vi "HandleObservationAsync.vi"(8 "error in (no error)":errorcluster, 10 "Acquisition.lvclass In":refnum<class "Acquisition.lvclass">, 11 "S4ACS_GUI in":refnum<class "S4ACS_GUI.lvclass">) -> (0 "error out":errorcluster, 2 "Acquisition.lvclass Out":refnum<class "Acquisition.lvclass">, 3 "S4ACS_GUI out":refnum<class "S4ACS_GUI.lvclass">)   [LabVIEW 2018, in "S4ACS_GUI.lvclass"]
uses:
  S4ACS_GUI.lvclass
  Acquisition/Acquisition.lvclass
  S4ACS_GUI.lvclass/S4ACS_GUI.ctl
  Instrument/Instrument.lvclass/Instrument.ctl
  Device/Optics/Optics.lvclass/Optics.ctl
  Device/Optics/Opt_Selector/Opt_Selector.lvclass
  C:/Users/observer/Desktop/Sparc4GUI/SPARC4_GUI/Device/Optics/Optics.lvclass
  Instrument/Instrument.lvclass
  StateMachine/State Machine.lvclass
  SyncBox/Sync Box.lvclass
  Trigger/Trigger.lvclass
  Channel/Channel.lvclass
  Device/Optics/Optics.lvclass
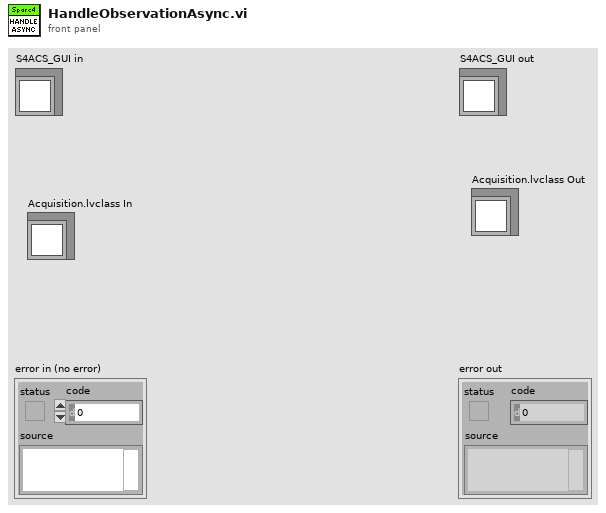
[diagram p1: front panel]
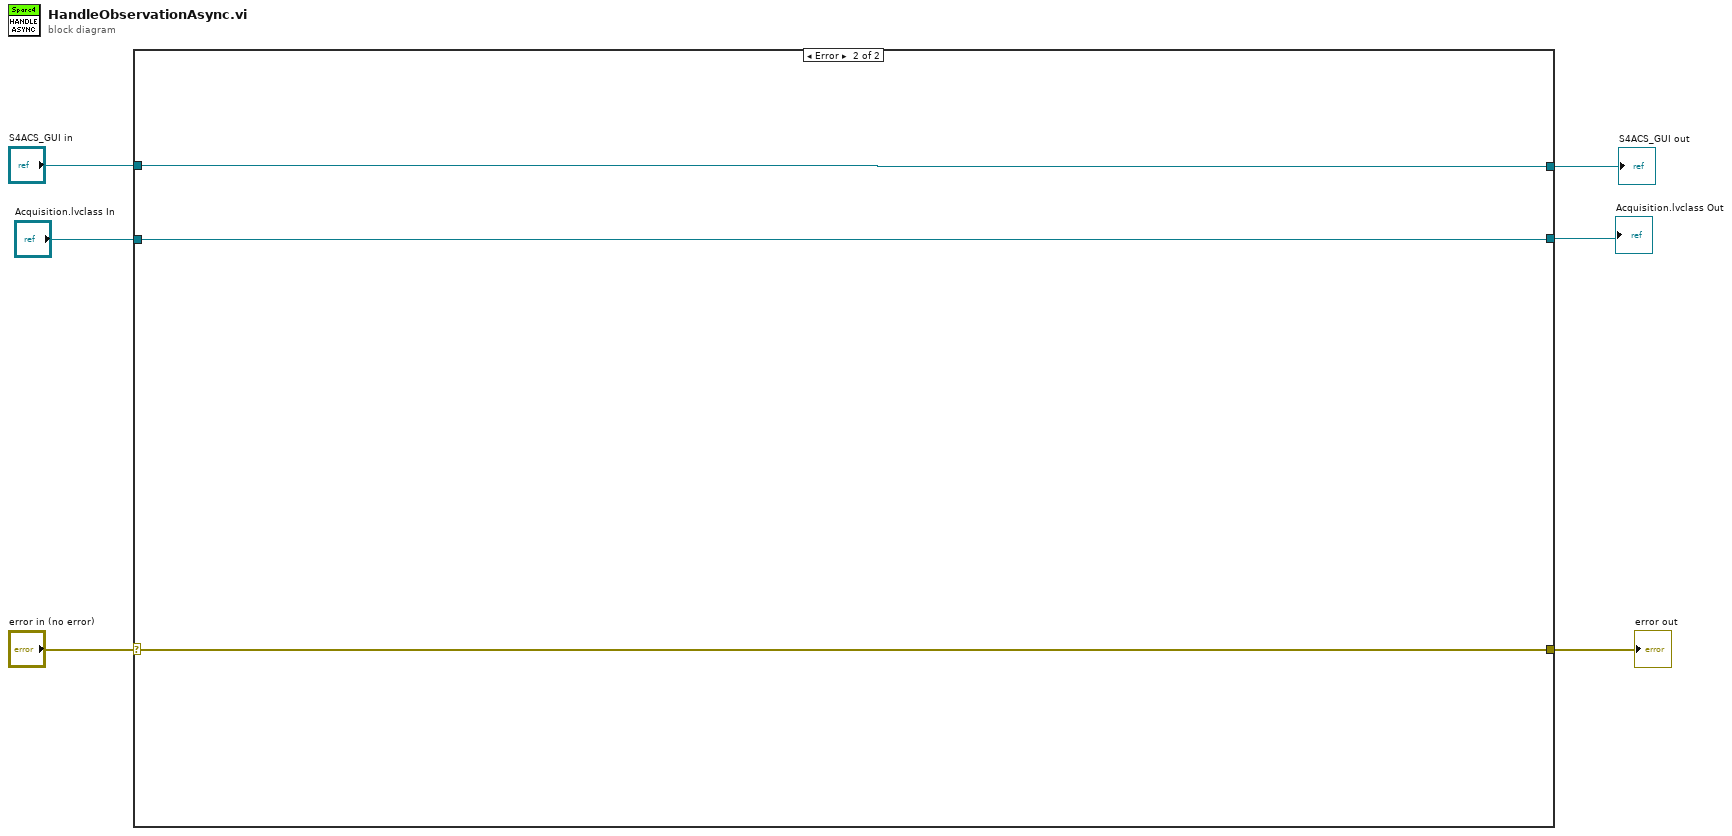
[diagram p0: block diagram]
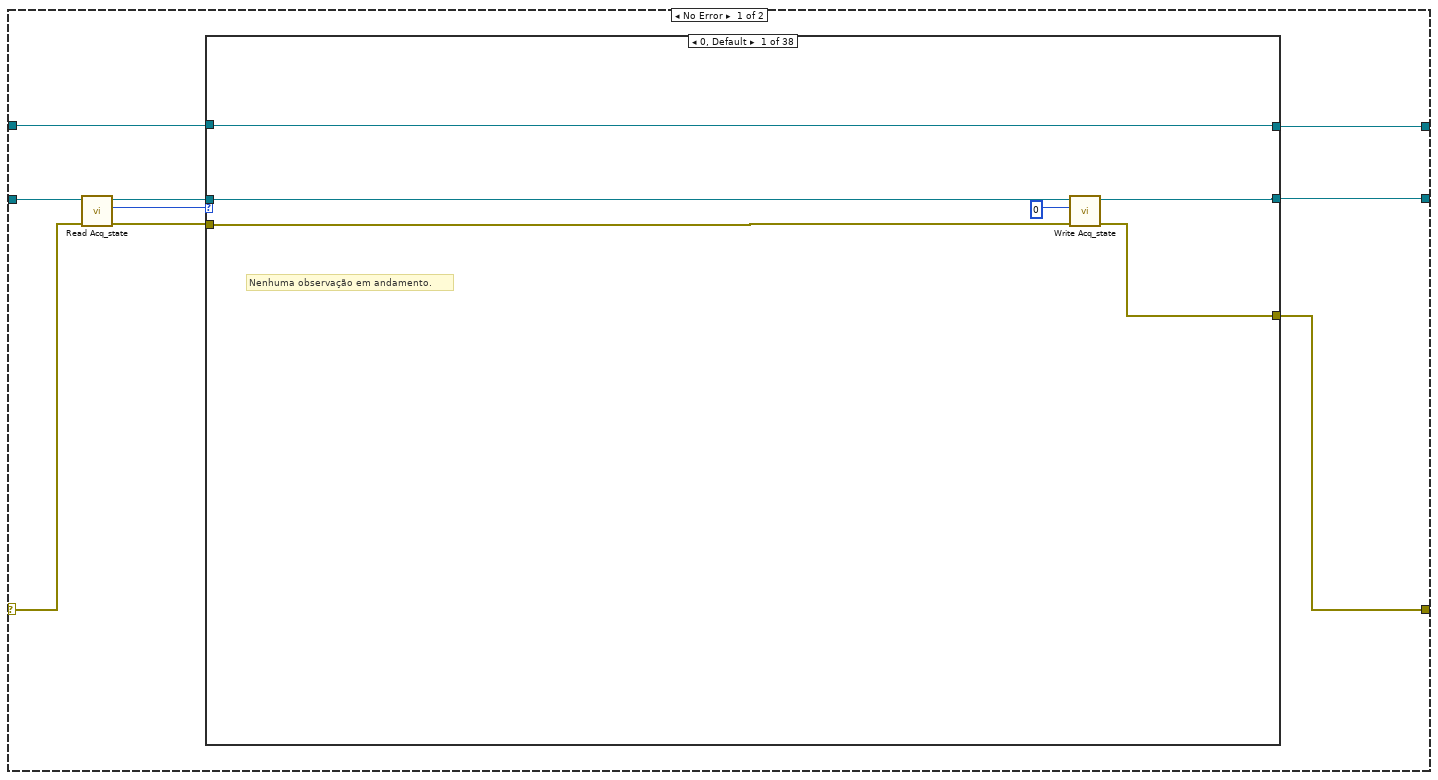
[diagram p2: hidden frame]
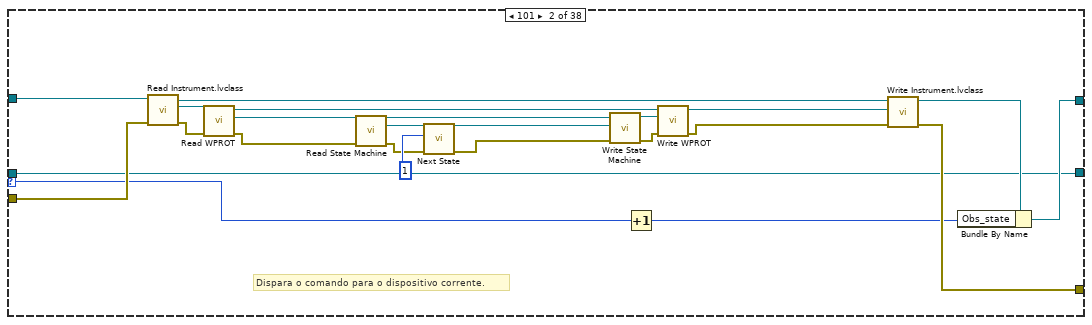
[diagram p3: hidden frame]
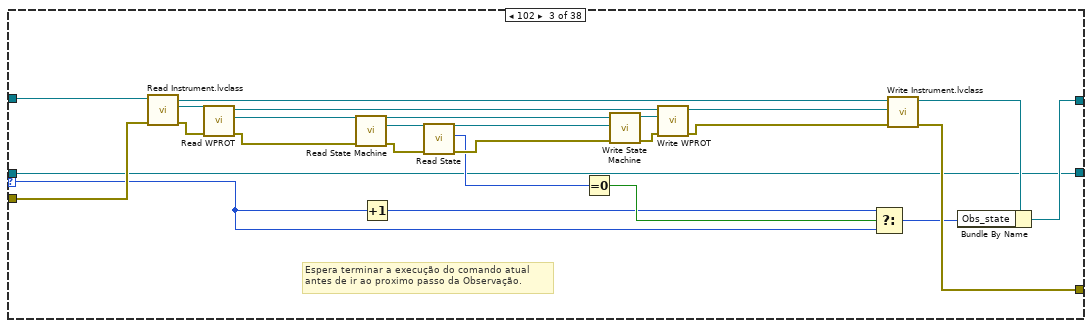
[diagram p4: hidden frame]
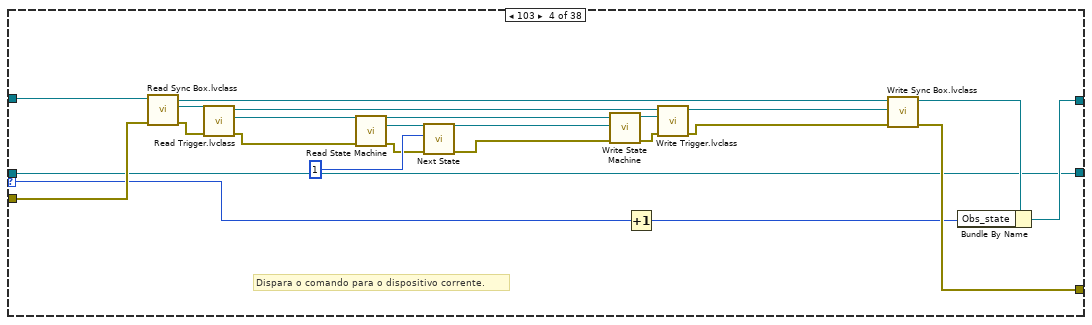
[diagram p5: hidden frame]
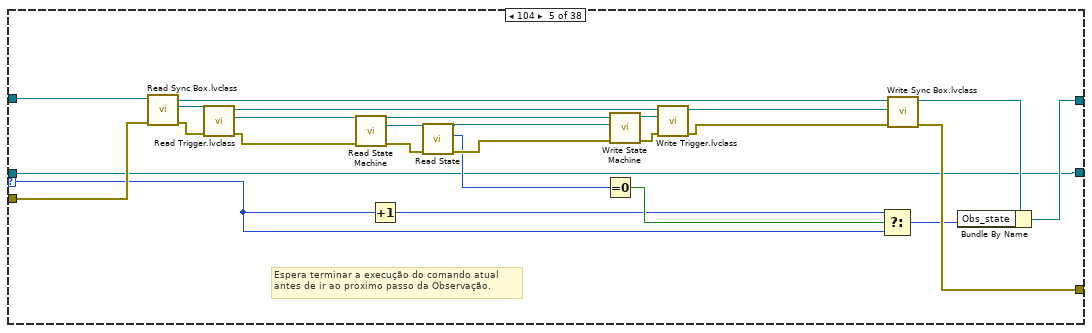
[diagram p6: hidden frame]
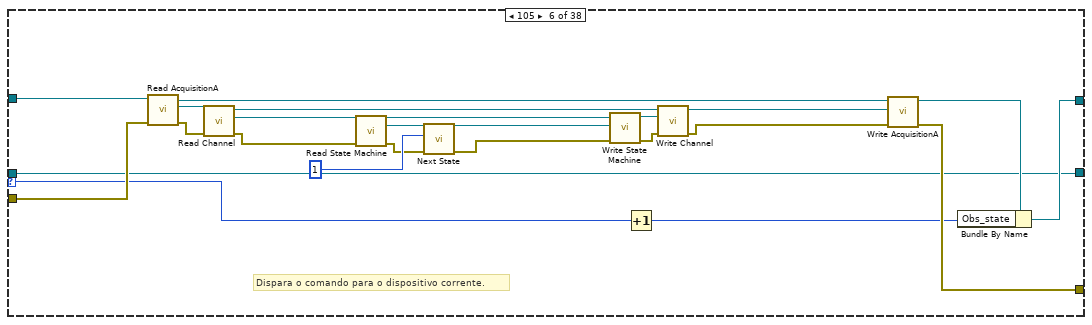
[diagram p7: hidden frame]
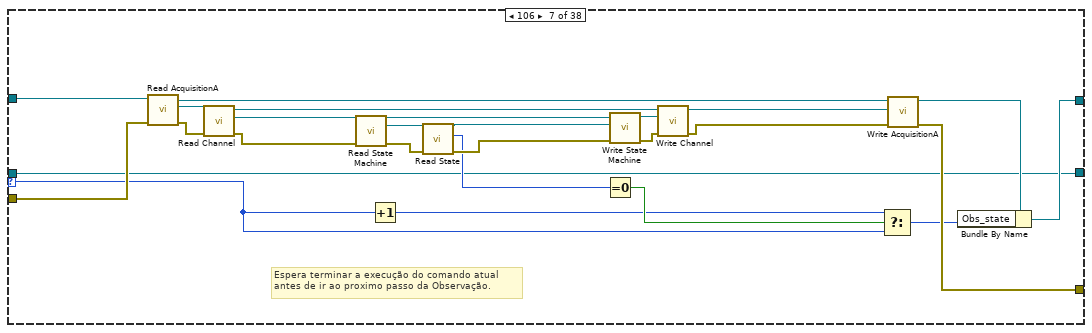
[diagram p8: hidden frame]
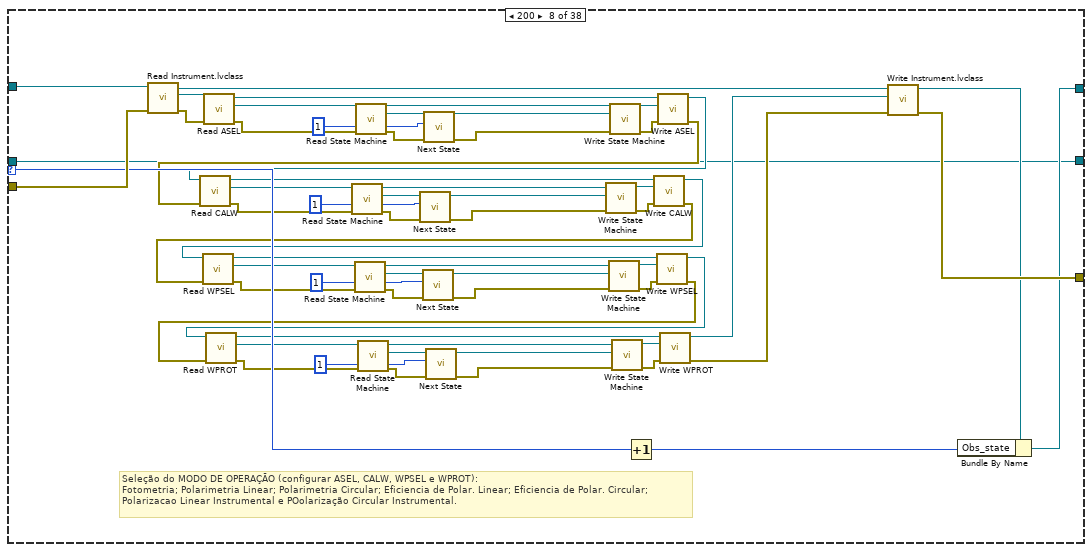
[diagram p9: hidden frame]
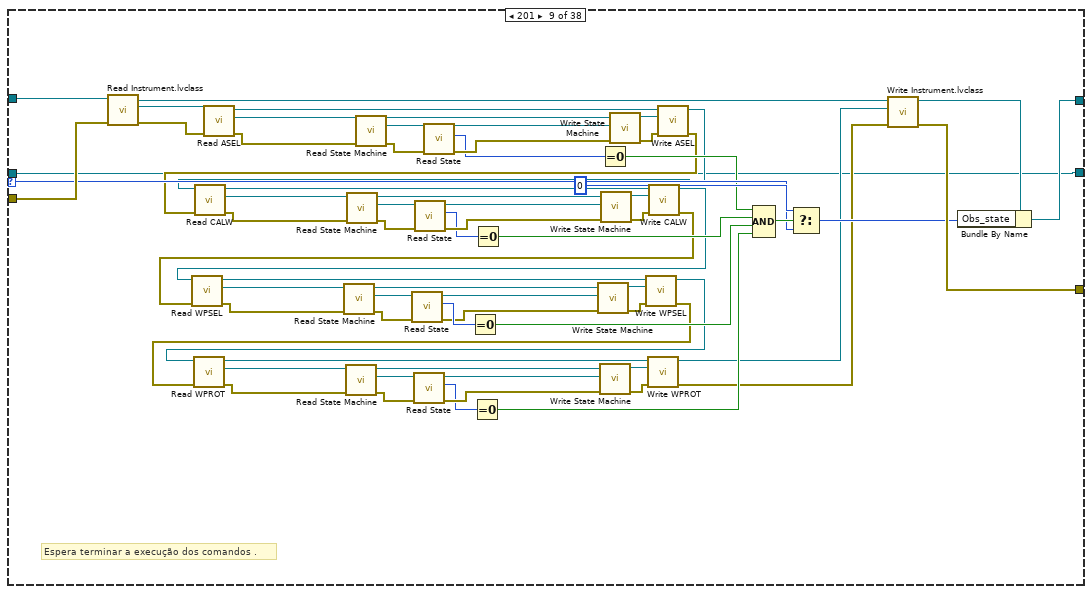
[diagram p10: hidden frame]
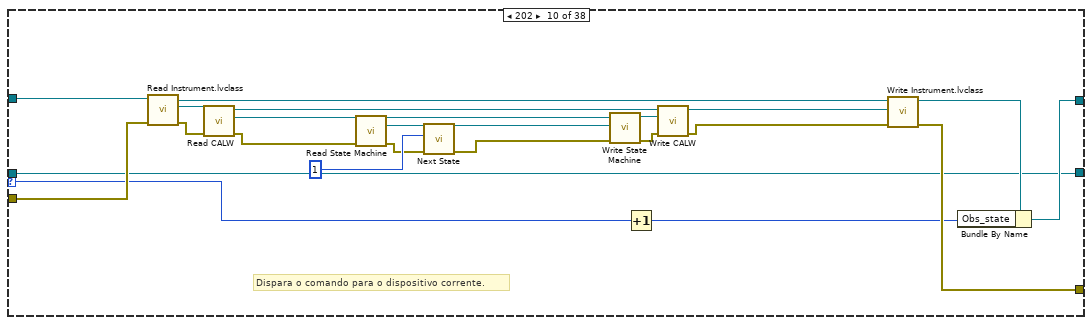
[diagram p11: hidden frame]
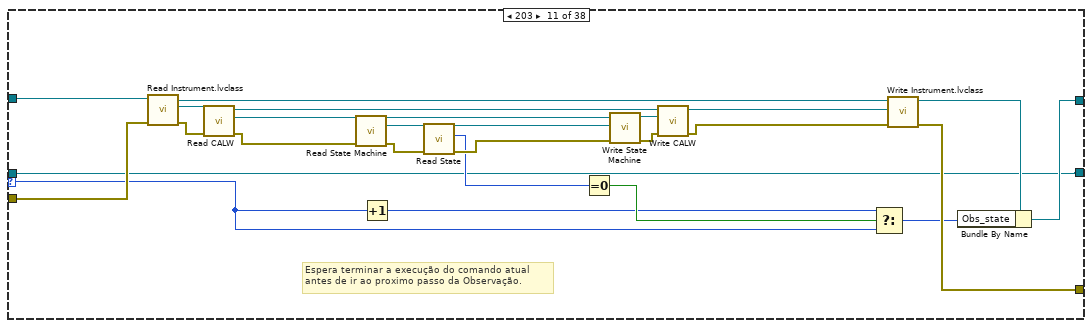
[diagram p12: hidden frame]
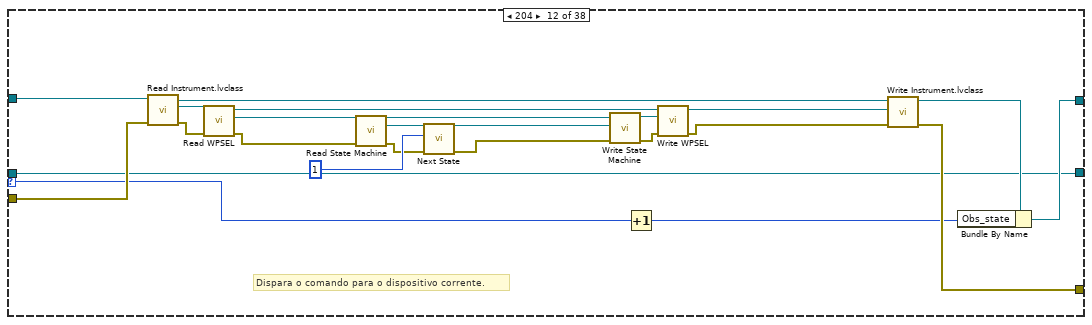
[diagram p13: hidden frame]
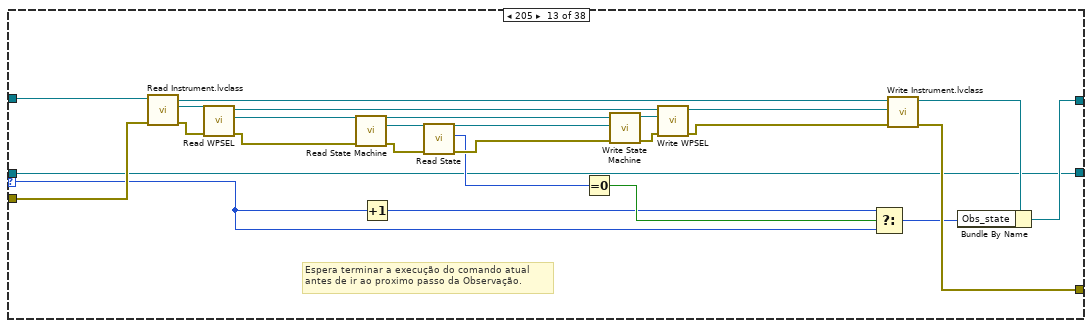
[diagram p14: hidden frame]
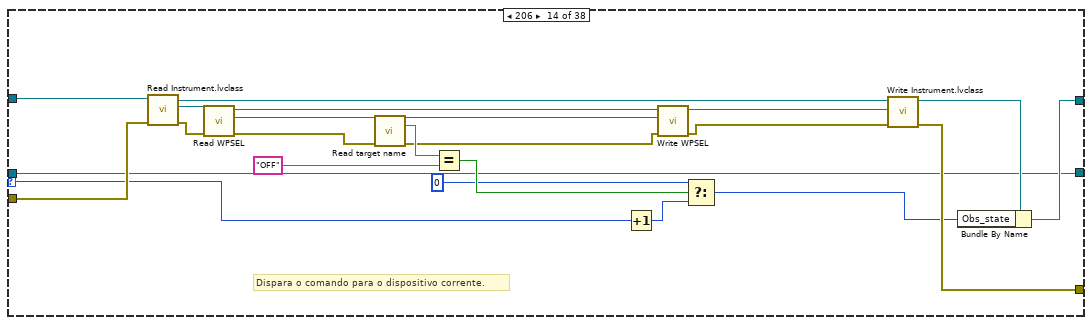
[diagram p15: hidden frame]
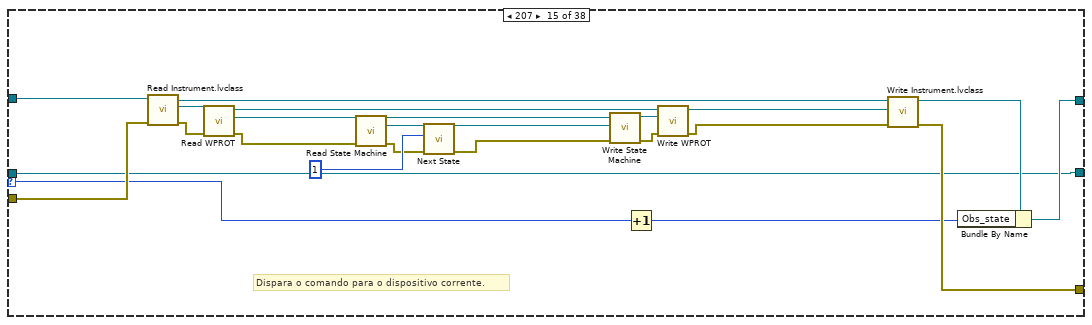
[diagram p16: hidden frame]
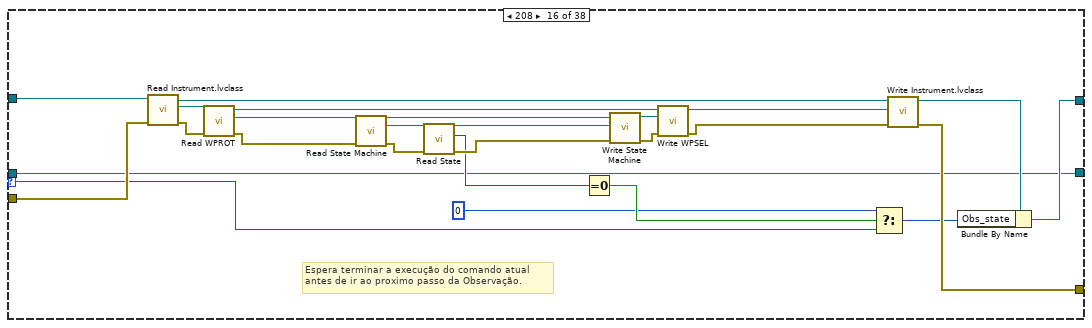
[diagram p17: hidden frame]
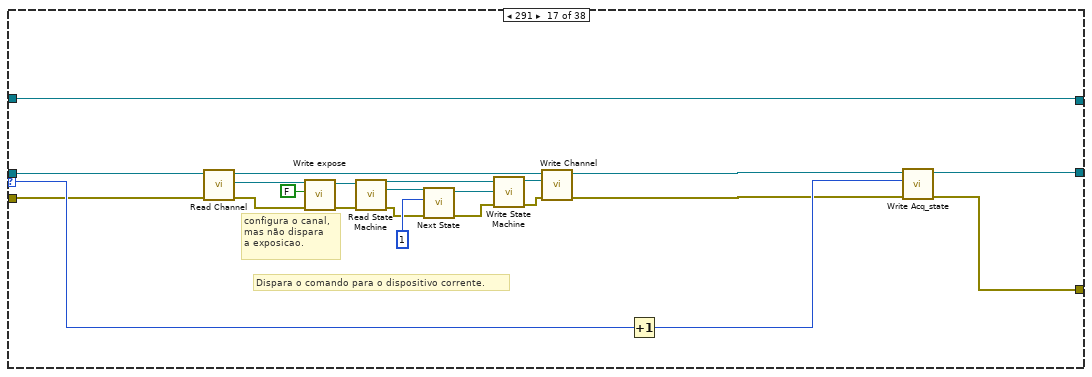
[diagram p18: hidden frame]
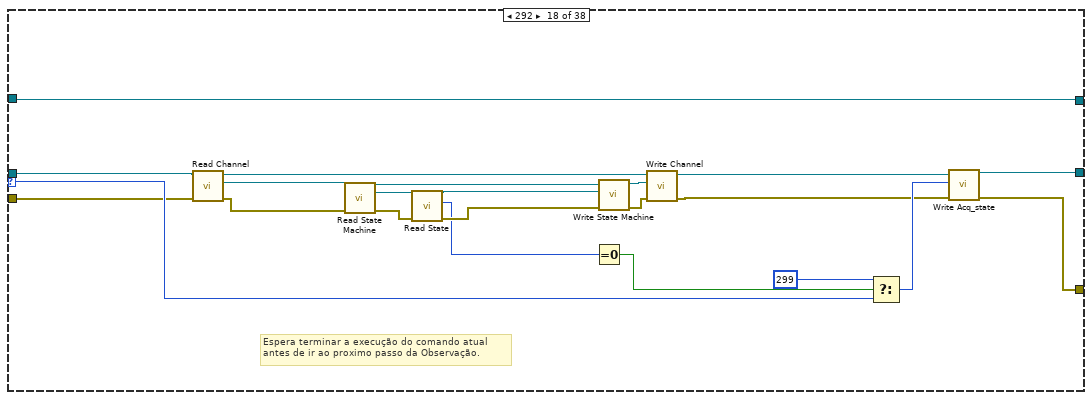
[diagram p19: hidden frame]
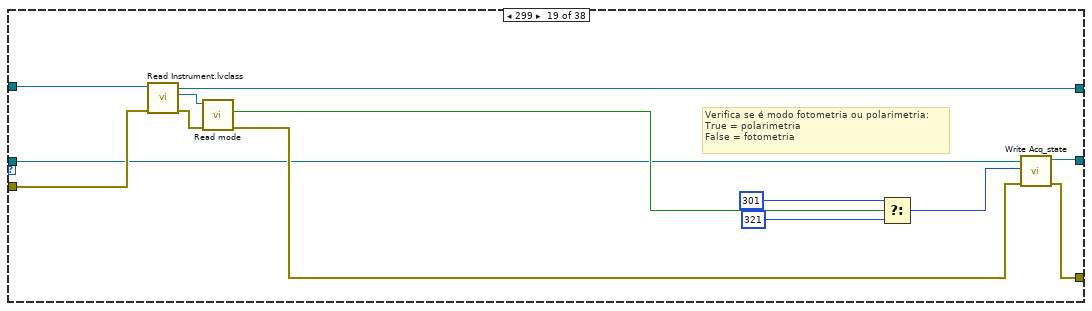
[diagram p20: hidden frame]
diagram:
  n1 = case shown="Error" "error in (no error)" {
    selector: "error in (no error)" -> [w9 w1155]
    tunnel: [w15 w1155] -> w5
    tunnel: [w14 w1154] -> w3
    tunnel: "S4ACS_GUI in" -> [w13 w1154]
    tunnel: "Acquisition.lvclass In" -> [w12 w1153]
    tunnel: [w7 w1153] -> w1
    frame No Error {
      n2 = call-dynamic "Read Acq_state.vi"("error in (no error)"=w9, "Acquisition in"=w12) -> ("error out"=w8:errorcluster, "Acq_state"=w10:u32, "Acquisition out"=w11:refnum<class "Acquisition.lvclass">)  [unwired: 7 in]
      n3 = case shown="0, Default" w10 {
        selector: w10 -> [_ w25 w48 w75 w98 w125 w148 w217 w281 w307 w330 w357 w380 w416 w430 w453 w492 w508 _ w570 w620 w644 w675 w718 w758 w774 w805 w845 w881 _ w931 w974 w1014 w1035 w1075 w1111 _ _]
        tunnel: w13 -> [w20 w39 w65 w89 w115 w139 w165 w231 w299 w321 w347 w371 w397 w420 w444 w470 w479 w506 w534 w572 w631 w657 w677 w730 w749 w787 w807 w857 w874 w903 w933 w986 w1002 w1037 w1087 w1104 w1135 w1152]
        tunnel: [w20 w23 w52 w73 w106 w123 w156 w215 w286 w305 w334 w355 w384 w415 w428 w457 w479 w506 w527 w537 w608 w643 w674 w712 w749 w773 w804 w844 w874 w903 w930 w973 w1002 w1029 w1074 w1104 w1135 w1152] -> w14
        tunnel: w8 -> [w19 w38 w64 w88 w114 w138 w164 w230 w298 w320 w346 w370 w396 w419 w443 w469 w483 w500 w533 w571 w630 w656 w676 w729 w751 w786 w806 w856 w878 w910 w932 w985 w1007 w1036 w1086 w1103 w1139 w1151]
        tunnel: [w16 w37 w63 w87 w113 w137 w163 w229 w297 w319 w345 w369 w395 w418 w442 w468 w477 w501 w523 w536 w610 w639 w670 w707 w745 w769 w799 w841 w872 w896 w925 w970 w1001 w1026 w1071 w1107 w1125 w1151] -> w15
        tunnel: w11 -> [w18 w22 w46 w72 w96 w122 w146 w172 w235 w304 w328 w354 w378 w404 w427 w451 w484 w507 w524 w539 w612 w638 w669 w709 w752 w768 w800 w834 w879 w909 w926 w969 w1008 w1024 w1064 w1102 w1140 w1150]
        tunnel: [w17 w22 w46 w72 w96 w122 w146 w172 w235 w304 w328 w354 w378 w404 w427 w451 w480 w502 w522 w535 w609 w640 w671 w708 w746 w772 w803 w842 w873 w897 w929 w972 w1006 w1025 w1072 w1109 w1131 w1150] -> w7
        frame 0, Default {
          # "Nenhuma observação em andamento."
          n4 = call-dynamic "Write Acq_state.vi"("error in (no error)"=w19, "Acq_state"=u32 0 ("Obs_state"), "Acquisition in"=w18) -> ("error out"=w16:errorcluster, "Acquisition out"=w17:refnum<class "Acquisition.lvclass">)  [unwired: 7 in]
        }
        frame 101 {
          # "Dispara o comando para o dispositivo corrente."
          n5 = call "Read Instrument.lvclass.vi"("error in (no error)"=w38, "S4ACS_GUI in"=w39) -> ("error out"=w44:errorcluster, "Instrument.lvclass"=w45:refnum<class "Instrument.lvclass">, "S4ACS_GUI out"=w41:refnum<class "S4ACS_GUI.lvclass">)  [unwired: 7 in]
          n6 = call "Read WPROT.vi"("error in (no error)"=w44, "Instrument in"=w45) -> ("error out"=w31:errorcluster, "Opt_Selector.lvclass"=w30:refnum<class "Opt_Selector.lvclass">, "Instrument out"=w43:refnum<class "Instrument.lvclass">)  [unwired: 7 in]
          n7 = call-dynamic "Read State Machine.vi"("error in (no error)"=w31, "Device in"=w30) -> ("error out"=w34:errorcluster, "State Machine.lvclass"=w36:refnum<class "State Machine.lvclass">, "Device out"=w28:refnum<class "Opt_Selector.lvclass">)  [unwired: 7 in]
          n8 = call "Next State.vi"("error in (no error)"=w34, "New_State"=1, "State Machine in"=w36) -> ("error out"=w33:errorcluster, "State Machine out"=w32:refnum<class "State Machine.lvclass">)  [unwired: 7 in]
          n9 = call-dynamic "Write State Machine.vi"("error in (no error)"=w33, "State Machine.lvclass"=w32, "Device in"=w28) -> ("error out"=w27:errorcluster, "Device out"=w29:refnum<class "Opt_Selector.lvclass">)  [unwired: 7 in]
          n10 = Increment(x=w25) -> (x+1=w24:u32)
          n11 = call "Write WPROT.vi"("error in (no error)"=w27, "Opt_Selector.lvclass"=w29, "Instrument in"=w43) -> ("error out"=w40:errorcluster, "Instrument out"=w42:refnum<class "Instrument.lvclass">)  [unwired: 7 in]
          n12 = call "Write Instrument.lvclass.vi"("error in (no error)"=w40, "Instrument.lvclass"=w42, "S4ACS_GUI in"=w41) -> ("error out"=w37:errorcluster, "S4ACS_GUI out"=w26:refnum<class "S4ACS_GUI.lvclass">)  [unwired: 7 in]
          n13 = Bundle By Name(cluster=w26, "Obs_state"=w24) -> (w23:refnum<class "S4ACS_GUI.lvclass">)
        }
        frame 102 {
          # "Espera terminar a execução do comando atual \nantes de ir ao proximo passo da Observação."
          n14 = call "Read Instrument.lvclass.vi"("error in (no error)"=w64, "S4ACS_GUI in"=w65) -> ("error out"=w70:errorcluster, "Instrument.lvclass"=w71:refnum<class "Instrument.lvclass">, "S4ACS_GUI out"=w67:refnum<class "S4ACS_GUI.lvclass">)  [unwired: 7 in]
          n15 = call "Read WPROT.vi"("error in (no error)"=w70, "Instrument in"=w71) -> ("error out"=w58:errorcluster, "Opt_Selector.lvclass"=w57:refnum<class "Opt_Selector.lvclass">, "Instrument out"=w69:refnum<class "Instrument.lvclass">)  [unwired: 7 in]
          n16 = call-dynamic "Read State Machine.vi"("error in (no error)"=w58, "Device in"=w57) -> ("error out"=w61:errorcluster, "State Machine.lvclass"=w62:refnum<class "State Machine.lvclass">, "Device out"=w55:refnum<class "Opt_Selector.lvclass">)  [unwired: 7 in]
          n17 = Increment(x=w48) -> (x+1=w47:u32)
          n18 = call-dynamic "Read State.vi"("error in (no error)"=w61, "State Machine in"=w62) -> ("error out"=w60:errorcluster, "State"=w50:i32, "State Machine out"=w59:refnum<class "State Machine.lvclass">)  [unwired: 7 in]
          n19 = Equal To 0?(x=w50) -> (x = 0?=w51:bool)
          n20 = call-dynamic "Write State Machine.vi"("error in (no error)"=w60, "State Machine.lvclass"=w59, "Device in"=w55) -> ("error out"=w54:errorcluster, "Device out"=w56:refnum<class "Opt_Selector.lvclass">)  [unwired: 7 in]
          n21 = call "Write WPROT.vi"("error in (no error)"=w54, "Opt_Selector.lvclass"=w56, "Instrument in"=w69) -> ("error out"=w66:errorcluster, "Instrument out"=w68:refnum<class "Instrument.lvclass">)  [unwired: 7 in]
          n22 = Select(t=w47, s=w51, f=w48) -> (s? t:f=w49:u32)
          n23 = call "Write Instrument.lvclass.vi"("error in (no error)"=w66, "Instrument.lvclass"=w68, "S4ACS_GUI in"=w67) -> ("error out"=w63:errorcluster, "S4ACS_GUI out"=w53:refnum<class "S4ACS_GUI.lvclass">)  [unwired: 7 in]
          n24 = Bundle By Name(cluster=w53, "Obs_state"=w49) -> (w52:refnum<class "S4ACS_GUI.lvclass">)
        }
        frame 103 {
          # "Dispara o comando para o dispositivo corrente."
          n25 = call-dynamic "Read Sync Box.lvclass.vi"("error in (no error)"=w88, "SPARC4_AC in"=w89) -> ("error out"=w94:errorcluster, "Sync Box.lvclass"=w95:refnum<class "Sync Box.lvclass">, "SPARC4_AC out"=w91:refnum<class "S4ACS_GUI.lvclass">)  [unwired: 7 in]
          n26 = call-dynamic "Read Trigger.lvclass.vi"("error in (no error)"=w94, "Sync Box in"=w95) -> ("error out"=w81:errorcluster, "Trigger.lvclass"=w80:refnum<class "Trigger.lvclass">, "Sync Box out"=w93:refnum<class "Sync Box.lvclass">)  [unwired: 7 in]
          n27 = call-dynamic "Read State Machine.vi"("error in (no error)"=w81, "Device in"=w80) -> ("error out"=w84:errorcluster, "State Machine.lvclass"=w86:refnum<class "State Machine.lvclass">, "Device out"=w78:refnum<class "Trigger.lvclass">)  [unwired: 7 in]
          n28 = call "Next State.vi"("error in (no error)"=w84, "New_State"=1, "State Machine in"=w86) -> ("error out"=w83:errorcluster, "State Machine out"=w82:refnum<class "State Machine.lvclass">)  [unwired: 7 in]
          n29 = call-dynamic "Write State Machine.vi"("error in (no error)"=w83, "State Machine.lvclass"=w82, "Device in"=w78) -> ("error out"=w77:errorcluster, "Device out"=w79:refnum<class "Trigger.lvclass">)  [unwired: 7 in]
          n30 = Increment(x=w75) -> (x+1=w74:u32)
          n31 = call-dynamic "Write Trigger.lvclass.vi"("error in (no error)"=w77, "Trigger.lvclass"=w79, "Sync Box in"=w93) -> ("error out"=w90:errorcluster, "Sync Box out"=w92:refnum<class "Sync Box.lvclass">)  [unwired: 7 in]
          n32 = call-dynamic "Write Sync Box.lvclass.vi"("error in (no error)"=w90, "Sync Box.lvclass"=w92, "SPARC4_AC in"=w91) -> ("error out"=w87:errorcluster, "SPARC4_AC out"=w76:refnum<class "S4ACS_GUI.lvclass">)  [unwired: 7 in]
          n33 = Bundle By Name(cluster=w76, "Obs_state"=w74) -> (w73:refnum<class "S4ACS_GUI.lvclass">)
        }
        frame 104 {
          # "Espera terminar a execução do comando atual \nantes de ir ao proximo passo da Observação."
          n34 = call-dynamic "Read Sync Box.lvclass.vi"("error in (no error)"=w114, "SPARC4_AC in"=w115) -> ("error out"=w120:errorcluster, "Sync Box.lvclass"=w121:refnum<class "Sync Box.lvclass">, "SPARC4_AC out"=w117:refnum<class "S4ACS_GUI.lvclass">)  [unwired: 7 in]
          n35 = call-dynamic "Read Trigger.lvclass.vi"("error in (no error)"=w120, "Sync Box in"=w121) -> ("error out"=w112:errorcluster, "Trigger.lvclass"=w111:refnum<class "Trigger.lvclass">, "Sync Box out"=w119:refnum<class "Sync Box.lvclass">)  [unwired: 7 in]
          n36 = call-dynamic "Read State Machine.vi"("error in (no error)"=w112, "Device in"=w111) -> ("error out"=w103:errorcluster, "State Machine.lvclass"=w105:refnum<class "State Machine.lvclass">, "Device out"=w109:refnum<class "Trigger.lvclass">)  [unwired: 7 in]
          n37 = Increment(x=w98) -> (x+1=w100:u32)
          n38 = call-dynamic "Read State.vi"("error in (no error)"=w103, "State Machine in"=w105) -> ("error out"=w102:errorcluster, "State"=w97:i32, "State Machine out"=w104:refnum<class "State Machine.lvclass">)  [unwired: 7 in]
          n39 = Equal To 0?(x=w97) -> (x = 0?=w101:bool)
          n40 = call-dynamic "Write State Machine.vi"("error in (no error)"=w102, "State Machine.lvclass"=w104, "Device in"=w109) -> ("error out"=w108:errorcluster, "Device out"=w110:refnum<class "Trigger.lvclass">)  [unwired: 7 in]
          n41 = call-dynamic "Write Trigger.lvclass.vi"("error in (no error)"=w108, "Trigger.lvclass"=w110, "Sync Box in"=w119) -> ("error out"=w116:errorcluster, "Sync Box out"=w118:refnum<class "Sync Box.lvclass">)  [unwired: 7 in]
          n42 = Select(t=w100, s=w101, f=w98) -> (s? t:f=w99:u32)
          n43 = call-dynamic "Write Sync Box.lvclass.vi"("error in (no error)"=w116, "Sync Box.lvclass"=w118, "SPARC4_AC in"=w117) -> ("error out"=w113:errorcluster, "SPARC4_AC out"=w107:refnum<class "S4ACS_GUI.lvclass">)  [unwired: 7 in]
          n44 = Bundle By Name(cluster=w107, "Obs_state"=w99) -> (w106:refnum<class "S4ACS_GUI.lvclass">)
        }
        frame 105 {
          # "Dispara o comando para o dispositivo corrente."
          n45 = call-dynamic "Read AcquisitionA.vi"("error in (no error)"=w138, "S4ACS_GUI in"=w139) -> ("error out"=w144:errorcluster, "Acquisition.lvclass"=w145:refnum<class "Acquisition.lvclass">, "S4ACS_GUI out"=w141:refnum<class "S4ACS_GUI.lvclass">)  [unwired: 7 in]
          n46 = call-dynamic "Read Channel.vi"("error in (no error)"=w144, "Acquisition in"=w145) -> ("error out"=w131:errorcluster, "Channel.lvclass"=w130:refnum<class "Channel.lvclass">, "Acquisition out"=w143:refnum<class "Acquisition.lvclass">)  [unwired: 7 in]
          n47 = call-dynamic "Read State Machine.vi"("error in (no error)"=w131, "Device in"=w130) -> ("error out"=w134:errorcluster, "State Machine.lvclass"=w136:refnum<class "State Machine.lvclass">, "Device out"=w128:refnum<class "Channel.lvclass">)  [unwired: 7 in]
          n48 = call "Next State.vi"("error in (no error)"=w134, "New_State"=1, "State Machine in"=w136) -> ("error out"=w133:errorcluster, "State Machine out"=w132:refnum<class "State Machine.lvclass">)  [unwired: 7 in]
          n49 = call-dynamic "Write State Machine.vi"("error in (no error)"=w133, "State Machine.lvclass"=w132, "Device in"=w128) -> ("error out"=w127:errorcluster, "Device out"=w129:refnum<class "Channel.lvclass">)  [unwired: 7 in]
          n50 = Increment(x=w125) -> (x+1=w124:u32)
          n51 = call-dynamic "Write Channel.vi"("error in (no error)"=w127, "Channel.lvclass"=w129, "Acquisition in"=w143) -> ("error out"=w140:errorcluster, "Acquisition out"=w142:refnum<class "Acquisition.lvclass">)  [unwired: 7 in]
          n52 = call-dynamic "Write AcquisitionA.vi"("error in (no error)"=w140, "Acquisition.lvclass"=w142, "S4ACS_GUI in"=w141) -> ("error out"=w137:errorcluster, "S4ACS_GUI out"=w126:refnum<class "S4ACS_GUI.lvclass">)  [unwired: 7 in]
          n53 = Bundle By Name(cluster=w126, "Obs_state"=w124) -> (w123:refnum<class "S4ACS_GUI.lvclass">)
        }
        frame 106 {
          # "Espera terminar a execução do comando atual \nantes de ir ao proximo passo da Observação."
          n54 = call-dynamic "Read AcquisitionA.vi"("error in (no error)"=w164, "S4ACS_GUI in"=w165) -> ("error out"=w170:errorcluster, "Acquisition.lvclass"=w171:refnum<class "Acquisition.lvclass">, "S4ACS_GUI out"=w167:refnum<class "S4ACS_GUI.lvclass">)  [unwired: 7 in]
          n55 = call-dynamic "Read Channel.vi"("error in (no error)"=w170, "Acquisition in"=w171) -> ("error out"=w162:errorcluster, "Channel.lvclass"=w161:refnum<class "Channel.lvclass">, "Acquisition out"=w169:refnum<class "Acquisition.lvclass">)  [unwired: 7 in]
          n56 = call-dynamic "Read State Machine.vi"("error in (no error)"=w162, "Device in"=w161) -> ("error out"=w153:errorcluster, "State Machine.lvclass"=w155:refnum<class "State Machine.lvclass">, "Device out"=w159:refnum<class "Channel.lvclass">)  [unwired: 7 in]
          n57 = Increment(x=w148) -> (x+1=w150:u32)
          n58 = call-dynamic "Read State.vi"("error in (no error)"=w153, "State Machine in"=w155) -> ("error out"=w152:errorcluster, "State"=w147:i32, "State Machine out"=w154:refnum<class "State Machine.lvclass">)  [unwired: 7 in]
          n59 = Equal To 0?(x=w147) -> (x = 0?=w151:bool)
          n60 = call-dynamic "Write State Machine.vi"("error in (no error)"=w152, "State Machine.lvclass"=w154, "Device in"=w159) -> ("error out"=w158:errorcluster, "Device out"=w160:refnum<class "Channel.lvclass">)  [unwired: 7 in]
          n61 = call-dynamic "Write Channel.vi"("error in (no error)"=w158, "Channel.lvclass"=w160, "Acquisition in"=w169) -> ("error out"=w166:errorcluster, "Acquisition out"=w168:refnum<class "Acquisition.lvclass">)  [unwired: 7 in]
          n62 = Select(t=w150, s=w151, f=w148) -> (s? t:f=w149:u32)
          n63 = call-dynamic "Write AcquisitionA.vi"("error in (no error)"=w166, "Acquisition.lvclass"=w168, "S4ACS_GUI in"=w167) -> ("error out"=w163:errorcluster, "S4ACS_GUI out"=w157:refnum<class "S4ACS_GUI.lvclass">)  [unwired: 7 in]
          n64 = Bundle By Name(cluster=w157, "Obs_state"=w149) -> (w156:refnum<class "S4ACS_GUI.lvclass">)
        }
        frame 200 {
          # "Seleção do MODO DE OPERAÇÃO (configurar ASEL, CALW, WPSEL e WPROT): \nFotometria; Polarimetria Linear; Polarimetria Circular; Eficiencia de Polar. Linear; Eficiencia de Polar. Circular;\nPolarizacao Linear Instrumental e POolarização Circular Instrumental."
          n65 = call "Read Instrument.lvclass.vi"("error in (no error)"=w230, "S4ACS_GUI in"=w231) -> ("error out"=w234:errorcluster, "Instrument.lvclass"=w194:refnum<class "Instrument.lvclass">, "S4ACS_GUI out"=w232:refnum<class "S4ACS_GUI.lvclass">)  [unwired: 7 in]
          n66 = call "Read ASEL.vi"("error in (no error)"=w234, "Instrument in"=w194) -> ("error out"=w223:errorcluster, "Opt_Selector.lvclass"=w222:refnum<class "Opt_Selector.lvclass">, "Instrument out"=w233:refnum<class "Instrument.lvclass">)  [unwired: 7 in]
          n67 = call-dynamic "Read State Machine.vi"("error in (no error)"=w223, "Device in"=w222) -> ("error out"=w226:errorcluster, "State Machine.lvclass"=w228:refnum<class "State Machine.lvclass">, "Device out"=w220:refnum<class "Opt_Selector.lvclass">)  [unwired: 7 in]
          n68 = call "Next State.vi"("error in (no error)"=w226, "New_State"=1, "State Machine in"=w228) -> ("error out"=w225:errorcluster, "State Machine out"=w224:refnum<class "State Machine.lvclass">)  [unwired: 7 in]
          n69 = call-dynamic "Write State Machine.vi"("error in (no error)"=w225, "State Machine.lvclass"=w224, "Device in"=w220) -> ("error out"=w219:errorcluster, "Device out"=w221:refnum<class "Opt_Selector.lvclass">)  [unwired: 7 in]
          n70 = Increment(x=w217) -> (x+1=w216:u32)
          n71 = call "Write ASEL.vi"("error in (no error)"=w219, "Opt_Selector.lvclass"=w221, "Instrument in"=w233) -> ("error out"=w175:errorcluster, "Instrument out"=w193:refnum<class "Instrument.lvclass">)  [unwired: 7 in]
          n72 = call "Read CALW.vi"("error in (no error)"=w175, "Instrument in"=w193) -> ("error out"=w210:errorcluster, "Opt_Selector.lvclass"=w211:refnum<class "Opt_Selector.lvclass">, "Instrument out"=w192:refnum<class "Instrument.lvclass">)  [unwired: 7 in]
          n73 = call-dynamic "Read State Machine.vi"("error in (no error)"=w210, "Device in"=w211) -> ("error out"=w207:errorcluster, "State Machine.lvclass"=w205:refnum<class "State Machine.lvclass">, "Device out"=w213:refnum<class "Opt_Selector.lvclass">)  [unwired: 7 in]
          n74 = call "Next State.vi"("error in (no error)"=w207, "New_State"=1, "State Machine in"=w205) -> ("error out"=w208:errorcluster, "State Machine out"=w209:refnum<class "State Machine.lvclass">)  [unwired: 7 in]
          n75 = call-dynamic "Write State Machine.vi"("error in (no error)"=w208, "State Machine.lvclass"=w209, "Device in"=w213) -> ("error out"=w214:errorcluster, "Device out"=w212:refnum<class "Opt_Selector.lvclass">)  [unwired: 7 in]
          n76 = call "Write CALW.vi"("error in (no error)"=w214, "Opt_Selector.lvclass"=w212, "Instrument in"=w192) -> ("error out"=w174:errorcluster, "Instrument out"=w191:refnum<class "Instrument.lvclass">)  [unwired: 7 in]
          n77 = call "Read WPSEL.vi"("error in (no error)"=w174, "Instrument in"=w191) -> ("error out"=w199:errorcluster, "Opt_Selector.lvclass"=w198:refnum<class "Opt_Selector.lvclass">, "Instrument out"=w190:refnum<class "Instrument.lvclass">)  [unwired: 7 in]
          n78 = call-dynamic "Read State Machine.vi"("error in (no error)"=w199, "Device in"=w198) -> ("error out"=w202:errorcluster, "State Machine.lvclass"=w204:refnum<class "State Machine.lvclass">, "Device out"=w196:refnum<class "Opt_Selector.lvclass">)  [unwired: 7 in]
          n79 = call "Next State.vi"("error in (no error)"=w202, "New_State"=1, "State Machine in"=w204) -> ("error out"=w201:errorcluster, "State Machine out"=w200:refnum<class "State Machine.lvclass">)  [unwired: 7 in]
          n80 = call-dynamic "Write State Machine.vi"("error in (no error)"=w201, "State Machine.lvclass"=w200, "Device in"=w196) -> ("error out"=w195:errorcluster, "Device out"=w197:refnum<class "Opt_Selector.lvclass">)  [unwired: 7 in]
          n81 = call "Write WPSEL.vi"("error in (no error)"=w195, "Opt_Selector.lvclass"=w197, "Instrument in"=w190) -> ("error out"=w173:errorcluster, "Instrument out"=w179:refnum<class "Instrument.lvclass">)  [unwired: 7 in]
          n82 = call "Read WPROT.vi"("error in (no error)"=w173, "Instrument in"=w179) -> ("error out"=w185:errorcluster, "Opt_Selector.lvclass"=w186:refnum<class "Opt_Selector.lvclass">, "Instrument out"=w178:refnum<class "Instrument.lvclass">)  [unwired: 7 in]
          n83 = call-dynamic "Read State Machine.vi"("error in (no error)"=w185, "Device in"=w186) -> ("error out"=w182:errorcluster, "State Machine.lvclass"=w180:refnum<class "State Machine.lvclass">, "Device out"=w188:refnum<class "Opt_Selector.lvclass">)  [unwired: 7 in]
          n84 = call "Next State.vi"("error in (no error)"=w182, "New_State"=1, "State Machine in"=w180) -> ("error out"=w183:errorcluster, "State Machine out"=w184:refnum<class "State Machine.lvclass">)  [unwired: 7 in]
          n85 = call-dynamic "Write State Machine.vi"("error in (no error)"=w183, "State Machine.lvclass"=w184, "Device in"=w188) -> ("error out"=w189:errorcluster, "Device out"=w187:refnum<class "Opt_Selector.lvclass">)  [unwired: 7 in]
          n86 = call "Write WPROT.vi"("error in (no error)"=w189, "Opt_Selector.lvclass"=w187, "Instrument in"=w178) -> ("error out"=w176:errorcluster, "Instrument out"=w177:refnum<class "Instrument.lvclass">)  [unwired: 7 in]
          n87 = call "Write Instrument.lvclass.vi"("error in (no error)"=w176, "Instrument.lvclass"=w177, "S4ACS_GUI in"=w232) -> ("error out"=w229:errorcluster, "S4ACS_GUI out"=w218:refnum<class "S4ACS_GUI.lvclass">)  [unwired: 7 in]
          n88 = Bundle By Name(cluster=w218, "Obs_state"=w216) -> (w215:refnum<class "S4ACS_GUI.lvclass">)
        }
        frame 201 {
          # "Espera terminar a execução dos comandos ."
          n89 = call "Read Instrument.lvclass.vi"("error in (no error)"=w298, "S4ACS_GUI in"=w299) -> ("error out"=w302:errorcluster, "Instrument.lvclass"=w303:refnum<class "Instrument.lvclass">, "S4ACS_GUI out"=w300:refnum<class "S4ACS_GUI.lvclass">)  [unwired: 7 in]
          n90 = call "Read ASEL.vi"("error in (no error)"=w302, "Instrument in"=w303) -> ("error out"=w292:errorcluster, "Opt_Selector.lvclass"=w291:refnum<class "Opt_Selector.lvclass">, "Instrument out"=w301:refnum<class "Instrument.lvclass">)  [unwired: 7 in]
          n91 = call-dynamic "Read State Machine.vi"("error in (no error)"=w292, "Device in"=w291) -> ("error out"=w295:errorcluster, "State Machine.lvclass"=w296:refnum<class "State Machine.lvclass">, "Device out"=w289:refnum<class "Opt_Selector.lvclass">)  [unwired: 7 in]
          n92 = call-dynamic "Read State.vi"("error in (no error)"=w295, "State Machine in"=w296) -> ("error out"=w294:errorcluster, "State"=w285:i32, "State Machine out"=w293:refnum<class "State Machine.lvclass">)  [unwired: 7 in]
          n93 = Equal To 0?(x=w285) -> (x = 0?=w280:bool)
          n94 = call-dynamic "Write State Machine.vi"("error in (no error)"=w294, "State Machine.lvclass"=w293, "Device in"=w289) -> ("error out"=w288:errorcluster, "Device out"=w290:refnum<class "Opt_Selector.lvclass">)  [unwired: 7 in]
          n95 = call "Write ASEL.vi"("error in (no error)"=w288, "Opt_Selector.lvclass"=w290, "Instrument in"=w301) -> ("error out"=w242:errorcluster, "Instrument out"=w243:refnum<class "Instrument.lvclass">)  [unwired: 7 in]
          n96 = call "Read CALW.vi"("error in (no error)"=w242, "Instrument in"=w243) -> ("error out"=w275:errorcluster, "Opt_Selector.lvclass"=w276:refnum<class "Opt_Selector.lvclass">, "Instrument out"=w246:refnum<class "Instrument.lvclass">)  [unwired: 7 in]
          n97 = call-dynamic "Read State Machine.vi"("error in (no error)"=w275, "Device in"=w276) -> ("error out"=w272:errorcluster, "State Machine.lvclass"=w271:refnum<class "State Machine.lvclass">, "Device out"=w278:refnum<class "Opt_Selector.lvclass">)  [unwired: 7 in]
          n98 = call-dynamic "Read State.vi"("error in (no error)"=w272, "State Machine in"=w271) -> ("error out"=w273:errorcluster, "State"=w270:i32, "State Machine out"=w274:refnum<class "State Machine.lvclass">)  [unwired: 7 in]
          n99 = Equal To 0?(x=w270) -> (x = 0?=w269:bool)
          n100 = call-dynamic "Write State Machine.vi"("error in (no error)"=w273, "State Machine.lvclass"=w274, "Device in"=w278) -> ("error out"=w279:errorcluster, "Device out"=w277:refnum<class "Opt_Selector.lvclass">)  [unwired: 7 in]
          n101 = call "Write CALW.vi"("error in (no error)"=w279, "Opt_Selector.lvclass"=w277, "Instrument in"=w246) -> ("error out"=w240:errorcluster, "Instrument out"=w241:refnum<class "Instrument.lvclass">)  [unwired: 7 in]
          n102 = call "Read WPSEL.vi"("error in (no error)"=w240, "Instrument in"=w241) -> ("error out"=w263:errorcluster, "Opt_Selector.lvclass"=w262:refnum<class "Opt_Selector.lvclass">, "Instrument out"=w245:refnum<class "Instrument.lvclass">)  [unwired: 7 in]
          n103 = call-dynamic "Read State Machine.vi"("error in (no error)"=w263, "Device in"=w262) -> ("error out"=w266:errorcluster, "State Machine.lvclass"=w267:refnum<class "State Machine.lvclass">, "Device out"=w260:refnum<class "Opt_Selector.lvclass">)  [unwired: 7 in]
          n104 = call-dynamic "Read State.vi"("error in (no error)"=w266, "State Machine in"=w267) -> ("error out"=w265:errorcluster, "State"=w268:i32, "State Machine out"=w264:refnum<class "State Machine.lvclass">)  [unwired: 7 in]
          n105 = Equal To 0?(x=w268) -> (x = 0?=w248:bool)
          n106 = call-dynamic "Write State Machine.vi"("error in (no error)"=w265, "State Machine.lvclass"=w264, "Device in"=w260) -> ("error out"=w259:errorcluster, "Device out"=w261:refnum<class "Opt_Selector.lvclass">)  [unwired: 7 in]
          n107 = call "Write WPSEL.vi"("error in (no error)"=w259, "Opt_Selector.lvclass"=w261, "Instrument in"=w245) -> ("error out"=w238:errorcluster, "Instrument out"=w239:refnum<class "Instrument.lvclass">)  [unwired: 7 in]
          n108 = call "Read WPROT.vi"("error in (no error)"=w238, "Instrument in"=w239) -> ("error out"=w254:errorcluster, "Opt_Selector.lvclass"=w255:refnum<class "Opt_Selector.lvclass">, "Instrument out"=w244:refnum<class "Instrument.lvclass">)  [unwired: 7 in]
          n109 = call-dynamic "Read State Machine.vi"("error in (no error)"=w254, "Device in"=w255) -> ("error out"=w251:errorcluster, "State Machine.lvclass"=w250:refnum<class "State Machine.lvclass">, "Device out"=w257:refnum<class "Opt_Selector.lvclass">)  [unwired: 7 in]
          n110 = call-dynamic "Read State.vi"("error in (no error)"=w251, "State Machine in"=w250) -> ("error out"=w252:errorcluster, "State"=w249:i32, "State Machine out"=w253:refnum<class "State Machine.lvclass">)  [unwired: 7 in]
          n111 = Equal To 0?(x=w249) -> (x = 0?=w247:bool)
          n112 = call-dynamic "Write State Machine.vi"("error in (no error)"=w252, "State Machine.lvclass"=w253, "Device in"=w257) -> ("error out"=w258:errorcluster, "Device out"=w256:refnum<class "Opt_Selector.lvclass">)  [unwired: 7 in]
          n113 = call "Write WPROT.vi"("error in (no error)"=w258, "Opt_Selector.lvclass"=w256, "Instrument in"=w244) -> ("error out"=w236:errorcluster, "Instrument out"=w237:refnum<class "Instrument.lvclass">)  [unwired: 7 in]
          n114 = Compound Arithmetic op=AND(w280, w269, w248, w247) -> (w282:bool)
          n115 = Select(t=u32 0, s=w282, f=w281) -> (s? t:f=w284:u32)
          n116 = call "Write Instrument.lvclass.vi"("error in (no error)"=w236, "Instrument.lvclass"=w237, "S4ACS_GUI in"=w300) -> ("error out"=w297:errorcluster, "S4ACS_GUI out"=w287:refnum<class "S4ACS_GUI.lvclass">)  [unwired: 7 in]
          n117 = Bundle By Name(cluster=w287, "Obs_state"=w284) -> (w286:refnum<class "S4ACS_GUI.lvclass">)
        }
        frame 202 {
          # "Dispara o comando para o dispositivo corrente."
          n118 = call "Read Instrument.lvclass.vi"("error in (no error)"=w320, "S4ACS_GUI in"=w321) -> ("error out"=w326:errorcluster, "Instrument.lvclass"=w327:refnum<class "Instrument.lvclass">, "S4ACS_GUI out"=w323:refnum<class "S4ACS_GUI.lvclass">)  [unwired: 7 in]
          n119 = call "Read CALW.vi"("error in (no error)"=w326, "Instrument in"=w327) -> ("error out"=w313:errorcluster, "Opt_Selector.lvclass"=w312:refnum<class "Opt_Selector.lvclass">, "Instrument out"=w325:refnum<class "Instrument.lvclass">)  [unwired: 7 in]
          n120 = call-dynamic "Read State Machine.vi"("error in (no error)"=w313, "Device in"=w312) -> ("error out"=w316:errorcluster, "State Machine.lvclass"=w318:refnum<class "State Machine.lvclass">, "Device out"=w310:refnum<class "Opt_Selector.lvclass">)  [unwired: 7 in]
          n121 = call "Next State.vi"("error in (no error)"=w316, "New_State"=1, "State Machine in"=w318) -> ("error out"=w315:errorcluster, "State Machine out"=w314:refnum<class "State Machine.lvclass">)  [unwired: 7 in]
          n122 = call-dynamic "Write State Machine.vi"("error in (no error)"=w315, "State Machine.lvclass"=w314, "Device in"=w310) -> ("error out"=w309:errorcluster, "Device out"=w311:refnum<class "Opt_Selector.lvclass">)  [unwired: 7 in]
          n123 = Increment(x=w307) -> (x+1=w306:u32)
          n124 = call "Write CALW.vi"("error in (no error)"=w309, "Opt_Selector.lvclass"=w311, "Instrument in"=w325) -> ("error out"=w322:errorcluster, "Instrument out"=w324:refnum<class "Instrument.lvclass">)  [unwired: 7 in]
          n125 = call "Write Instrument.lvclass.vi"("error in (no error)"=w322, "Instrument.lvclass"=w324, "S4ACS_GUI in"=w323) -> ("error out"=w319:errorcluster, "S4ACS_GUI out"=w308:refnum<class "S4ACS_GUI.lvclass">)  [unwired: 7 in]
          n126 = Bundle By Name(cluster=w308, "Obs_state"=w306) -> (w305:refnum<class "S4ACS_GUI.lvclass">)
        }
        frame 203 {
          # "Espera terminar a execução do comando atual \nantes de ir ao proximo passo da Observação."
          n127 = call "Read Instrument.lvclass.vi"("error in (no error)"=w346, "S4ACS_GUI in"=w347) -> ("error out"=w352:errorcluster, "Instrument.lvclass"=w353:refnum<class "Instrument.lvclass">, "S4ACS_GUI out"=w349:refnum<class "S4ACS_GUI.lvclass">)  [unwired: 7 in]
          n128 = call "Read CALW.vi"("error in (no error)"=w352, "Instrument in"=w353) -> ("error out"=w340:errorcluster, "Opt_Selector.lvclass"=w339:refnum<class "Opt_Selector.lvclass">, "Instrument out"=w351:refnum<class "Instrument.lvclass">)  [unwired: 7 in]
          n129 = call-dynamic "Read State Machine.vi"("error in (no error)"=w340, "Device in"=w339) -> ("error out"=w343:errorcluster, "State Machine.lvclass"=w344:refnum<class "State Machine.lvclass">, "Device out"=w337:refnum<class "Opt_Selector.lvclass">)  [unwired: 7 in]
          n130 = Increment(x=w330) -> (x+1=w329:u32)
          n131 = call-dynamic "Read State.vi"("error in (no error)"=w343, "State Machine in"=w344) -> ("error out"=w342:errorcluster, "State"=w332:i32, "State Machine out"=w341:refnum<class "State Machine.lvclass">)  [unwired: 7 in]
          n132 = Equal To 0?(x=w332) -> (x = 0?=w333:bool)
          n133 = call-dynamic "Write State Machine.vi"("error in (no error)"=w342, "State Machine.lvclass"=w341, "Device in"=w337) -> ("error out"=w336:errorcluster, "Device out"=w338:refnum<class "Opt_Selector.lvclass">)  [unwired: 7 in]
          n134 = call "Write CALW.vi"("error in (no error)"=w336, "Opt_Selector.lvclass"=w338, "Instrument in"=w351) -> ("error out"=w348:errorcluster, "Instrument out"=w350:refnum<class "Instrument.lvclass">)  [unwired: 7 in]
          n135 = Select(t=w329, s=w333, f=w330) -> (s? t:f=w331:u32)
          n136 = call "Write Instrument.lvclass.vi"("error in (no error)"=w348, "Instrument.lvclass"=w350, "S4ACS_GUI in"=w349) -> ("error out"=w345:errorcluster, "S4ACS_GUI out"=w335:refnum<class "S4ACS_GUI.lvclass">)  [unwired: 7 in]
          n137 = Bundle By Name(cluster=w335, "Obs_state"=w331) -> (w334:refnum<class "S4ACS_GUI.lvclass">)
        }
        frame 204 {
          # "Dispara o comando para o dispositivo corrente."
          n138 = call "Read Instrument.lvclass.vi"("error in (no error)"=w370, "S4ACS_GUI in"=w371) -> ("error out"=w376:errorcluster, "Instrument.lvclass"=w377:refnum<class "Instrument.lvclass">, "S4ACS_GUI out"=w373:refnum<class "S4ACS_GUI.lvclass">)  [unwired: 7 in]
          n139 = call "Read WPSEL.vi"("error in (no error)"=w376, "Instrument in"=w377) -> ("error out"=w363:errorcluster, "Opt_Selector.lvclass"=w362:refnum<class "Opt_Selector.lvclass">, "Instrument out"=w375:refnum<class "Instrument.lvclass">)  [unwired: 7 in]
          n140 = call-dynamic "Read State Machine.vi"("error in (no error)"=w363, "Device in"=w362) -> ("error out"=w366:errorcluster, "State Machine.lvclass"=w368:refnum<class "State Machine.lvclass">, "Device out"=w360:refnum<class "Opt_Selector.lvclass">)  [unwired: 7 in]
          n141 = call "Next State.vi"("error in (no error)"=w366, "New_State"=1, "State Machine in"=w368) -> ("error out"=w365:errorcluster, "State Machine out"=w364:refnum<class "State Machine.lvclass">)  [unwired: 7 in]
          n142 = call-dynamic "Write State Machine.vi"("error in (no error)"=w365, "State Machine.lvclass"=w364, "Device in"=w360) -> ("error out"=w359:errorcluster, "Device out"=w361:refnum<class "Opt_Selector.lvclass">)  [unwired: 7 in]
          n143 = Increment(x=w357) -> (x+1=w356:u32)
          n144 = call "Write WPSEL.vi"("error in (no error)"=w359, "Opt_Selector.lvclass"=w361, "Instrument in"=w375) -> ("error out"=w372:errorcluster, "Instrument out"=w374:refnum<class "Instrument.lvclass">)  [unwired: 7 in]
          n145 = call "Write Instrument.lvclass.vi"("error in (no error)"=w372, "Instrument.lvclass"=w374, "S4ACS_GUI in"=w373) -> ("error out"=w369:errorcluster, "S4ACS_GUI out"=w358:refnum<class "S4ACS_GUI.lvclass">)  [unwired: 7 in]
          n146 = Bundle By Name(cluster=w358, "Obs_state"=w356) -> (w355:refnum<class "S4ACS_GUI.lvclass">)
        }
        frame 205 {
          # "Espera terminar a execução do comando atual \nantes de ir ao proximo passo da Observação."
          n147 = call "Read Instrument.lvclass.vi"("error in (no error)"=w396, "S4ACS_GUI in"=w397) -> ("error out"=w402:errorcluster, "Instrument.lvclass"=w403:refnum<class "Instrument.lvclass">, "S4ACS_GUI out"=w399:refnum<class "S4ACS_GUI.lvclass">)  [unwired: 7 in]
          n148 = call "Read WPSEL.vi"("error in (no error)"=w402, "Instrument in"=w403) -> ("error out"=w390:errorcluster, "Opt_Selector.lvclass"=w389:refnum<class "Opt_Selector.lvclass">, "Instrument out"=w401:refnum<class "Instrument.lvclass">)  [unwired: 7 in]
          n149 = call-dynamic "Read State Machine.vi"("error in (no error)"=w390, "Device in"=w389) -> ("error out"=w393:errorcluster, "State Machine.lvclass"=w394:refnum<class "State Machine.lvclass">, "Device out"=w387:refnum<class "Opt_Selector.lvclass">)  [unwired: 7 in]
          n150 = Increment(x=w380) -> (x+1=w379:u32)
          n151 = call-dynamic "Read State.vi"("error in (no error)"=w393, "State Machine in"=w394) -> ("error out"=w392:errorcluster, "State"=w382:i32, "State Machine out"=w391:refnum<class "State Machine.lvclass">)  [unwired: 7 in]
          n152 = Equal To 0?(x=w382) -> (x = 0?=w383:bool)
          n153 = call-dynamic "Write State Machine.vi"("error in (no error)"=w392, "State Machine.lvclass"=w391, "Device in"=w387) -> ("error out"=w386:errorcluster, "Device out"=w388:refnum<class "Opt_Selector.lvclass">)  [unwired: 7 in]
          n154 = call "Write WPSEL.vi"("error in (no error)"=w386, "Opt_Selector.lvclass"=w388, "Instrument in"=w401) -> ("error out"=w398:errorcluster, "Instrument out"=w400:refnum<class "Instrument.lvclass">)  [unwired: 7 in]
          n155 = Select(t=w379, s=w383, f=w380) -> (s? t:f=w381:u32)
          n156 = call "Write Instrument.lvclass.vi"("error in (no error)"=w398, "Instrument.lvclass"=w400, "S4ACS_GUI in"=w399) -> ("error out"=w395:errorcluster, "S4ACS_GUI out"=w385:refnum<class "S4ACS_GUI.lvclass">)  [unwired: 7 in]
          n157 = Bundle By Name(cluster=w385, "Obs_state"=w381) -> (w384:refnum<class "S4ACS_GUI.lvclass">)
        }
        frame 206 {
          # "Dispara o comando para o dispositivo corrente."
          n158 = call "Read Instrument.lvclass.vi"("error in (no error)"=w419, "S4ACS_GUI in"=w420) -> ("error out"=w425:errorcluster, "Instrument.lvclass"=w426:refnum<class "Instrument.lvclass">, "S4ACS_GUI out"=w422:refnum<class "S4ACS_GUI.lvclass">)  [unwired: 7 in]
          n159 = call "Read WPSEL.vi"("error in (no error)"=w425, "Instrument in"=w426) -> ("error out"=w413:errorcluster, "Opt_Selector.lvclass"=w414:refnum<class "Opt_Selector.lvclass">, "Instrument out"=w424:refnum<class "Instrument.lvclass">)  [unwired: 7 in]
          n160 = call "Read target name.vi"("error in (no error)"=w413, "Optics in"=w414) -> ("error out"=w407:errorcluster, "target name"=w412:string, "Optics out"=w406:refnum<class "Opt_Selector.lvclass">)  [unwired: 7 in]
          n161 = Equal?(x=w412, y="OFF") -> (x = y?=w410:bool)
          n162 = Increment(x=w416) -> (x+1=w408:u32)
          n163 = call "Write WPSEL.vi"("error in (no error)"=w407, "Opt_Selector.lvclass"=w406, "Instrument in"=w424) -> ("error out"=w421:errorcluster, "Instrument out"=w423:refnum<class "Instrument.lvclass">)  [unwired: 7 in]
          n164 = Select(t=u32 0, s=w410, f=w408) -> (s? t:f=w405:u32)
          n165 = call "Write Instrument.lvclass.vi"("error in (no error)"=w421, "Instrument.lvclass"=w423, "S4ACS_GUI in"=w422) -> ("error out"=w418:errorcluster, "S4ACS_GUI out"=w417:refnum<class "S4ACS_GUI.lvclass">)  [unwired: 7 in]
          n166 = Bundle By Name(cluster=w417, "Obs_state"=w405) -> (w415:refnum<class "S4ACS_GUI.lvclass">)
        }
        frame 207 {
          # "Dispara o comando para o dispositivo corrente."
          n167 = call "Read Instrument.lvclass.vi"("error in (no error)"=w443, "S4ACS_GUI in"=w444) -> ("error out"=w449:errorcluster, "Instrument.lvclass"=w450:refnum<class "Instrument.lvclass">, "S4ACS_GUI out"=w446:refnum<class "S4ACS_GUI.lvclass">)  [unwired: 7 in]
          n168 = call "Read WPROT.vi"("error in (no error)"=w449, "Instrument in"=w450) -> ("error out"=w436:errorcluster, "Opt_Selector.lvclass"=w435:refnum<class "Opt_Selector.lvclass">, "Instrument out"=w448:refnum<class "Instrument.lvclass">)  [unwired: 7 in]
          n169 = call-dynamic "Read State Machine.vi"("error in (no error)"=w436, "Device in"=w435) -> ("error out"=w439:errorcluster, "State Machine.lvclass"=w441:refnum<class "State Machine.lvclass">, "Device out"=w433:refnum<class "Opt_Selector.lvclass">)  [unwired: 7 in]
          n170 = call "Next State.vi"("error in (no error)"=w439, "New_State"=1, "State Machine in"=w441) -> ("error out"=w438:errorcluster, "State Machine out"=w437:refnum<class "State Machine.lvclass">)  [unwired: 7 in]
          n171 = call-dynamic "Write State Machine.vi"("error in (no error)"=w438, "State Machine.lvclass"=w437, "Device in"=w433) -> ("error out"=w432:errorcluster, "Device out"=w434:refnum<class "Opt_Selector.lvclass">)  [unwired: 7 in]
          n172 = Increment(x=w430) -> (x+1=w429:u32)
          n173 = call "Write WPROT.vi"("error in (no error)"=w432, "Opt_Selector.lvclass"=w434, "Instrument in"=w448) -> ("error out"=w445:errorcluster, "Instrument out"=w447:refnum<class "Instrument.lvclass">)  [unwired: 7 in]
          n174 = call "Write Instrument.lvclass.vi"("error in (no error)"=w445, "Instrument.lvclass"=w447, "S4ACS_GUI in"=w446) -> ("error out"=w442:errorcluster, "S4ACS_GUI out"=w431:refnum<class "S4ACS_GUI.lvclass">)  [unwired: 7 in]
          n175 = Bundle By Name(cluster=w431, "Obs_state"=w429) -> (w428:refnum<class "S4ACS_GUI.lvclass">)
        }
        frame 208 {
          # "Espera terminar a execução do comando atual \nantes de ir ao proximo passo da Observação."
          n176 = call "Read Instrument.lvclass.vi"("error in (no error)"=w469, "S4ACS_GUI in"=w470) -> ("error out"=w475:errorcluster, "Instrument.lvclass"=w476:refnum<class "Instrument.lvclass">, "S4ACS_GUI out"=w472:refnum<class "S4ACS_GUI.lvclass">)  [unwired: 7 in]
          n177 = call "Read WPROT.vi"("error in (no error)"=w475, "Instrument in"=w476) -> ("error out"=w463:errorcluster, "Opt_Selector.lvclass"=w462:refnum<class "Opt_Selector.lvclass">, "Instrument out"=w474:refnum<class "Instrument.lvclass">)  [unwired: 7 in]
          n178 = call-dynamic "Read State Machine.vi"("error in (no error)"=w463, "Device in"=w462) -> ("error out"=w466:errorcluster, "State Machine.lvclass"=w467:refnum<class "State Machine.lvclass">, "Device out"=w460:refnum<class "Opt_Selector.lvclass">)  [unwired: 7 in]
          n179 = call-dynamic "Read State.vi"("error in (no error)"=w466, "State Machine in"=w467) -> ("error out"=w465:errorcluster, "State"=w455:i32, "State Machine out"=w464:refnum<class "State Machine.lvclass">)  [unwired: 7 in]
          n180 = Equal To 0?(x=w455) -> (x = 0?=w456:bool)
          n181 = call-dynamic "Write State Machine.vi"("error in (no error)"=w465, "State Machine.lvclass"=w464, "Device in"=w460) -> ("error out"=w459:errorcluster, "Device out"=w461:refnum<class "Opt_Selector.lvclass">)  [unwired: 7 in]
          n182 = call "Write WPSEL.vi"("error in (no error)"=w459, "Opt_Selector.lvclass"=w461, "Instrument in"=w474) -> ("error out"=w471:errorcluster, "Instrument out"=w473:refnum<class "Instrument.lvclass">)  [unwired: 7 in]
          n183 = Select(t=u32 0, s=w456, f=w453) -> (s? t:f=w454:u32)
          n184 = call "Write Instrument.lvclass.vi"("error in (no error)"=w471, "Instrument.lvclass"=w473, "S4ACS_GUI in"=w472) -> ("error out"=w468:errorcluster, "S4ACS_GUI out"=w458:refnum<class "S4ACS_GUI.lvclass">)  [unwired: 7 in]
          n185 = Bundle By Name(cluster=w458, "Obs_state"=w454) -> (w457:refnum<class "S4ACS_GUI.lvclass">)
        }
        frame 291 {
          # "configura o canal,\nmas não dispara\na exposicao."
          # "Dispara o comando para o dispositivo corrente."
          n186 = call-dynamic "Read Channel.vi"("error in (no error)"=w483, "Acquisition in"=w484) -> ("error out"=w489:errorcluster, "Channel.lvclass"=w491:refnum<class "Channel.lvclass">, "Acquisition out"=w499:refnum<class "Acquisition.lvclass">)  [unwired: 7 in]
          n187 = call-dynamic "Write expose.vi"("error in (no error)"=w489, "expose"=FALSE, "Channel in"=w491) -> ("error out"=w488:errorcluster, "Channel out"=w490:refnum<class "Channel.lvclass">)  [unwired: 7 in]
          n188 = call-dynamic "Read State Machine.vi"("error in (no error)"=w488, "Device in"=w490) -> ("error out"=w496:errorcluster, "State Machine.lvclass"=w498:refnum<class "State Machine.lvclass">, "Device out"=w494:refnum<class "Channel.lvclass">)  [unwired: 7 in]
          n189 = call "Next State.vi"("error in (no error)"=w496, "New_State"=1, "State Machine in"=w498) -> ("error out"=w485:errorcluster, "State Machine out"=w486:refnum<class "State Machine.lvclass">)  [unwired: 7 in]
          n190 = call-dynamic "Write State Machine.vi"("error in (no error)"=w485, "State Machine.lvclass"=w486, "Device in"=w494) -> ("error out"=w493:errorcluster, "Device out"=w495:refnum<class "Channel.lvclass">)  [unwired: 7 in]
          n191 = call-dynamic "Write Channel.vi"("error in (no error)"=w493, "Channel.lvclass"=w495, "Acquisition in"=w499) -> ("error out"=w478:errorcluster, "Acquisition out"=w481:refnum<class "Acquisition.lvclass">)  [unwired: 7 in]
          n192 = Increment(x=w492) -> (x+1=w482:u32)
          n193 = call-dynamic "Write Acq_state.vi"("error in (no error)"=w478, "Acq_state"=w482, "Acquisition in"=w481) -> ("error out"=w477:errorcluster, "Acquisition out"=w480:refnum<class "Acquisition.lvclass">)  [unwired: 7 in]
        }
        frame 292 {
          # "Espera terminar a execução do comando atual \nantes de ir ao proximo passo da Observação."
          n194 = call-dynamic "Read Channel.vi"("error in (no error)"=w500, "Acquisition in"=w507) -> ("error out"=w520:errorcluster, "Channel.lvclass"=w519:refnum<class "Channel.lvclass">, "Acquisition out"=w521:refnum<class "Acquisition.lvclass">)  [unwired: 7 in]
          n195 = call-dynamic "Read State Machine.vi"("error in (no error)"=w520, "Device in"=w519) -> ("error out"=w513:errorcluster, "State Machine.lvclass"=w515:refnum<class "State Machine.lvclass">, "Device out"=w517:refnum<class "Channel.lvclass">)  [unwired: 7 in]
          n196 = call-dynamic "Read State.vi"("error in (no error)"=w513, "State Machine in"=w515) -> ("error out"=w512:errorcluster, "State"=w510:i32, "State Machine out"=w514:refnum<class "State Machine.lvclass">)  [unwired: 7 in]
          n197 = Equal To 0?(x=w510) -> (x = 0?=w511:bool)
          n198 = call-dynamic "Write State Machine.vi"("error in (no error)"=w512, "State Machine.lvclass"=w514, "Device in"=w517) -> ("error out"=w516:errorcluster, "Device out"=w518:refnum<class "Channel.lvclass">)  [unwired: 7 in]
          n199 = call-dynamic "Write Channel.vi"("error in (no error)"=w516, "Channel.lvclass"=w518, "Acquisition in"=w521) -> ("error out"=w504:errorcluster, "Acquisition out"=w503:refnum<class "Acquisition.lvclass">)  [unwired: 7 in]
          n200 = Select(t=u32 299, s=w511, f=w508) -> (s? t:f=w505:u32)
          n201 = call-dynamic "Write Acq_state.vi"("error in (no error)"=w504, "Acq_state"=w505, "Acquisition in"=w503) -> ("error out"=w501:errorcluster, "Acquisition out"=w502:refnum<class "Acquisition.lvclass">)  [unwired: 7 in]
        }
        frame 299 {
          # "Verifica se é modo fotometria ou polarimetria:\nTrue = polarimetria\nFalse = fotometria"
          n202 = call "Read Instrument.lvclass.vi"("error in (no error)"=w533, "S4ACS_GUI in"=w534) -> ("error out"=w530:errorcluster, "Instrument.lvclass"=w531:refnum<class "Instrument.lvclass">, "S4ACS_GUI out"=w527:refnum<class "S4ACS_GUI.lvclass">)  [unwired: 7 in]
          n203 = call-dynamic "Read mode.vi"("error in (no error)"=w530, "Instrument in"=w531) -> ("error out"=w525:errorcluster, "mode"=w529:bool)  [unwired: 7 in, 1 out]
          n204 = Select(t=u32 301, s=w529, f=u32 321 ("t")) -> (s? t:f=w526:u32)
          n205 = call-dynamic "Write Acq_state.vi"("error in (no error)"=w525, "Acq_state"=w526, "Acquisition in"=w524) -> ("error out"=w523:errorcluster, "Acquisition out"=w522:refnum<class "Acquisition.lvclass">)  [unwired: 7 in]
        }
        frame 301 {
          n206 = call "Read Instrument.lvclass.vi"("error in (no error)"=w571, "S4ACS_GUI in"=w572) -> ("error out"=w575:errorcluster, "Instrument.lvclass"=w576:refnum<class "Instrument.lvclass">, "S4ACS_GUI out"=w573:refnum<class "S4ACS_GUI.lvclass">)  [unwired: 7 in]
          n207 = call "Read WPROT.vi"("error in (no error)"=w575, "Instrument in"=w576) -> ("error out"=w568:errorcluster, "Opt_Selector.lvclass"=w569:refnum<class "Opt_Selector.lvclass">, "Instrument out"=w574:refnum<class "Instrument.lvclass">)  [unwired: 7 in]
          n208 = call-dynamic "getTargetPos.vi"("error in (no error)"=w568, "Opt_Selector in"=w569) -> ("error out"=w567:errorcluster, "Target Pos"=w547:u16, "Opt_Selector out"=w566:refnum<class "Opt_Selector.lvclass">)  [unwired: 7 in]
          n209 = Build Array(-1.0 ("element"), 0.0 ("element"), 22.5 ("element"), 45.0 ("element"), 67.5 ("element"), 90.0 ("element"), 112.5 ("element"), 135.0 ("element"), 157.5 ("element"), 180.0 ("element"), 202.5 ("element"), 225.0 ("element"), 247.5 ("element"), 270.0 ("element"), 292.5 ("element"), 315.0 ("element"), 337.5 ("element")) -> (w559:dbl[])
          n210 = Index Array(array=w559, index=w547) -> (element=w546:dbl)
          n211 = case shown="1..16" w547 {
            selector: w547 -> [_ w599]
            tunnel: w574 -> [w584 w587]
            tunnel: [w584 w587] -> w542
            tunnel: [w581 w586] -> w541
            tunnel: w570 -> [_ w601]
            tunnel: [u32 311 w600] -> w540
            tunnel: w567 -> [w582 w595]
            tunnel: w566 -> [w583 w594]
            tunnel: w546 -> [_ w589]
            tunnel: [w579 w588] -> w543
            frame 0, Default {
              # "Verifica os ciclos"
              # "Recupera a sequencia anterior para o caso \nde repetição da sequencia (sem precisar clicar \nnas posicoes desejadas novamente)."
              n212 = call-dynamic "Read sequencia_ant.vi"("error in (no error)"=w582, "Opt_Selector in"=w583) -> ("error out"=w578:errorcluster, "sequencia_ant"=w577:u16, "Opt_Selector out"=w580:refnum<class "Opt_Selector.lvclass">)  [unwired: 7 in]
              n213 = call-dynamic "Write sequencia.vi"("error in (no error)"=w578, "sequencia"=w577, "Opt_Selector in"=w580) -> ("error out"=w581:errorcluster, "Opt_Selector out"=w579:refnum<class "Opt_Selector.lvclass">)  [unwired: 7 in]
            }
            frame 1..16 {
              n214 = Number To Decimal String(number=w599) -> (decimal integer string=w598:string)  [unwired: 1 in]
              n215 = Concatenate Strings("WP" ("string"), w598) -> (w596:string)
              n216 = call "Write target name.vi"("error in (no error)"=w595, "target name"=w596, "Optics in"=w594) -> ("error out"=w592:errorcluster, "Optics out"=w593:refnum<class "Opt_Selector.lvclass">)  [unwired: 7 in]
              n217 = call "Write target.vi"("error in (no error)"=w592, "target"=w589, "Optics in"=w593) -> ("error out"=w591:errorcluster, "Optics out"=w590:refnum<class "Opt_Selector.lvclass">)  [unwired: 7 in]
              n218 = call-dynamic "Read State Machine.vi"("error in (no error)"=w591, "Device in"=w590) -> ("error out"=w605:errorcluster, "State Machine.lvclass"=w607:refnum<class "State Machine.lvclass">, "Device out"=w602:refnum<class "Opt_Selector.lvclass">)  [unwired: 7 in]
              n219 = Increment(x=w601) -> (x+1=w600:u32)
              n220 = call "Next State.vi"("error in (no error)"=w605, "New_State"=1, "State Machine in"=w607) -> ("error out"=w604:errorcluster, "State Machine out"=w603:refnum<class "State Machine.lvclass">)  [unwired: 7 in]
              n221 = call-dynamic "Write State Machine.vi"("error in (no error)"=w604, "State Machine.lvclass"=w603, "Device in"=w602) -> ("error out"=w586:errorcluster, "Device out"=w588:refnum<class "Opt_Selector.lvclass">)  [unwired: 7 in]
            }
          }
          n222 = call "Write WPROT.vi"("error in (no error)"=w541, "Opt_Selector.lvclass"=w543, "Instrument in"=w542) -> ("error out"=w545:errorcluster, "Instrument out"=w544:refnum<class "Instrument.lvclass">)  [unwired: 7 in]
          n223 = call "Write Instrument.lvclass.vi"("error in (no error)"=w545, "Instrument.lvclass"=w544, "S4ACS_GUI in"=w573) -> ("error out"=w538:errorcluster, "S4ACS_GUI out"=w537:refnum<class "S4ACS_GUI.lvclass">)  [unwired: 7 in]
          n224 = call-dynamic "Write Acq_state.vi"("error in (no error)"=w538, "Acq_state"=w540, "Acquisition in"=w539) -> ("error out"=w536:errorcluster, "Acquisition out"=w535:refnum<class "Acquisition.lvclass">)  [unwired: 7 in]
        }
        frame 302 {
          # "TESTE: 1 x 20ms = 0.02s de pausa entre \nposições do waveplate."
          # "Espera terminar o movimento para a posição \"target\" do waveplate\nantes de ir para o estado de pausa."
          n225 = call "Read Instrument.lvclass.vi"("error in (no error)"=w630, "S4ACS_GUI in"=w631) -> ("error out"=w636:errorcluster, "Instrument.lvclass"=w637:refnum<class "Instrument.lvclass">, "S4ACS_GUI out"=w633:refnum<class "S4ACS_GUI.lvclass">)  [unwired: 7 in]
          n226 = call "Read WPROT.vi"("error in (no error)"=w636, "Instrument in"=w637) -> ("error out"=w627:errorcluster, "Opt_Selector.lvclass"=w626:refnum<class "Opt_Selector.lvclass">, "Instrument out"=w635:refnum<class "Instrument.lvclass">)  [unwired: 7 in]
          n227 = call-dynamic "Read State Machine.vi"("error in (no error)"=w627, "Device in"=w626) -> ("error out"=w628:errorcluster, "State Machine.lvclass"=w629:refnum<class "State Machine.lvclass">, "Device out"=w624:refnum<class "Opt_Selector.lvclass">)  [unwired: 7 in]
          n228 = Increment(x=w620) -> (x+1=w619:u32)
          n229 = call-dynamic "Read State.vi"("error in (no error)"=w628, "State Machine in"=w629) -> ("error out"=w614:errorcluster, "State"=w621:i32, "State Machine out"=w618:refnum<class "State Machine.lvclass">)  [unwired: 7 in]
          n230 = Equal To 0?(x=w621) -> (x = 0?=w622:bool)
          n231 = call-dynamic "Write Timer.vi"("error in (no error)"=w614, "Timer"=u32 1, "State Machine in"=w618) -> ("error out"=w615:errorcluster, "State Machine out"=w617:refnum<class "State Machine.lvclass">)  [unwired: 7 in]
          n232 = call-dynamic "Write State Machine.vi"("error in (no error)"=w615, "State Machine.lvclass"=w617, "Device in"=w624) -> ("error out"=w623:errorcluster, "Device out"=w625:refnum<class "Opt_Selector.lvclass">)  [unwired: 7 in]
          n233 = call "Write WPROT.vi"("error in (no error)"=w623, "Opt_Selector.lvclass"=w625, "Instrument in"=w635) -> ("error out"=w632:errorcluster, "Instrument out"=w634:refnum<class "Instrument.lvclass">)  [unwired: 7 in]
          n234 = Select(t=w619, s=w622, f=w620) -> (s? t:f=w613:u32)
          n235 = call "Write Instrument.lvclass.vi"("error in (no error)"=w632, "Instrument.lvclass"=w634, "S4ACS_GUI in"=w633) -> ("error out"=w611:errorcluster, "S4ACS_GUI out"=w608:refnum<class "S4ACS_GUI.lvclass">)  [unwired: 7 in]
          n236 = call-dynamic "Write Acq_state.vi"("error in (no error)"=w611, "Acq_state"=w613, "Acquisition in"=w612) -> ("error out"=w610:errorcluster, "Acquisition out"=w609:refnum<class "Acquisition.lvclass">)  [unwired: 7 in]
        }
        frame 303 {
          # "Espera terminar a pausa carregada no Timer"
          n237 = call "Read Instrument.lvclass.vi"("error in (no error)"=w656, "S4ACS_GUI in"=w657) -> ("error out"=w662:errorcluster, "Instrument.lvclass"=w663:refnum<class "Instrument.lvclass">, "S4ACS_GUI out"=w659:refnum<class "S4ACS_GUI.lvclass">)  [unwired: 7 in]
          n238 = call "Read WPROT.vi"("error in (no error)"=w662, "Instrument in"=w663) -> ("error out"=w655:errorcluster, "Opt_Selector.lvclass"=w654:refnum<class "Opt_Selector.lvclass">, "Instrument out"=w661:refnum<class "Instrument.lvclass">)  [unwired: 7 in]
          n239 = call-dynamic "Read State Machine.vi"("error in (no error)"=w655, "Device in"=w654) -> ("error out"=w647:errorcluster, "State Machine.lvclass"=w648:refnum<class "State Machine.lvclass">, "Device out"=w652:refnum<class "Opt_Selector.lvclass">)  [unwired: 7 in]
          n240 = Increment(x=w644) -> (x+1=w649:u32)
          n241 = call "Verify Timer.vi"("error in (no error)"=w647, "State Machine in"=w648) -> ("error out"=w645:errorcluster, "timeout"=w650:bool, "State Machine out"=w646:refnum<class "State Machine.lvclass">)  [unwired: 7 in]
          n242 = call-dynamic "Write State Machine.vi"("error in (no error)"=w645, "State Machine.lvclass"=w646, "Device in"=w652) -> ("error out"=w651:errorcluster, "Device out"=w653:refnum<class "Opt_Selector.lvclass">)  [unwired: 7 in]
          n243 = call "Write WPROT.vi"("error in (no error)"=w651, "Opt_Selector.lvclass"=w653, "Instrument in"=w661) -> ("error out"=w658:errorcluster, "Instrument out"=w660:refnum<class "Instrument.lvclass">)  [unwired: 7 in]
          n244 = call "Write Instrument.lvclass.vi"("error in (no error)"=w658, "Instrument.lvclass"=w660, "S4ACS_GUI in"=w659) -> ("error out"=w642:errorcluster, "S4ACS_GUI out"=w643:refnum<class "S4ACS_GUI.lvclass">)  [unwired: 7 in]
          n245 = Select(t=w649, s=w650, f=w644) -> (s? t:f=w641:u32)
          n246 = call-dynamic "Write Acq_state.vi"("error in (no error)"=w642, "Acq_state"=w641, "Acquisition in"=w638) -> ("error out"=w639:errorcluster, "Acquisition out"=w640:refnum<class "Acquisition.lvclass">)  [unwired: 7 in]
        }
        frame 304 {
          # "SyncBox ocupado?"
          n247 = call-dynamic "Read Sync Box.lvclass.vi"("error in (no error)"=w676, "SPARC4_AC in"=w677) -> ("error out"=w667:errorcluster, "Sync Box.lvclass"=w668:refnum<class "Sync Box.lvclass">, "SPARC4_AC out"=w679:refnum<class "S4ACS_GUI.lvclass">)  [unwired: 7 in]
          n248 = call-dynamic "Read busy.vi"("error in (no error)"=w667, "Sync Box in"=w668) -> ("error out"=w664:errorcluster, "busy"=w666:bool, "Sync Box out"=w665:refnum<class "Sync Box.lvclass">)  [unwired: 7 in]
          n249 = case shown="False" w666 {
            tunnel: w664 -> [w703 w704]
            tunnel: [w684 w705] -> w680
            tunnel: [w682 w704] -> w678
            tunnel: w675 -> [w693 w706]
            tunnel: w665 -> [w687 w705]
            tunnel: [w686 w706] -> w673
            frame False {
              # "configura delays do syncBox"
              # "Dispara o comando para o dispositivo corrente."
              n250 = call-dynamic "Read Trigger.lvclass.vi"("error in (no error)"=w703, "Sync Box in"=w687) -> ("error out"=w698:errorcluster, "Trigger.lvclass"=w697:refnum<class "Trigger.lvclass">, "Sync Box out"=w702:refnum<class "Sync Box.lvclass">)  [unwired: 7 in]
              n251 = call-dynamic "Read State Machine.vi"("error in (no error)"=w698, "Device in"=w697) -> ("error out"=w699:errorcluster, "State Machine.lvclass"=w701:refnum<class "State Machine.lvclass">, "Device out"=w695:refnum<class "Trigger.lvclass">)  [unwired: 7 in]
              n252 = call "Next State.vi"("error in (no error)"=w699, "New_State"=10, "State Machine in"=w701) -> ("error out"=w689:errorcluster, "State Machine out"=w691:refnum<class "State Machine.lvclass">)  [unwired: 7 in]
              n253 = call-dynamic "Write Timer.vi"("error in (no error)"=w689, "Timer"=u32 5, "State Machine in"=w691) -> ("error out"=w688:errorcluster, "State Machine out"=w690:refnum<class "State Machine.lvclass">)  [unwired: 7 in]
              n254 = call-dynamic "Write State Machine.vi"("error in (no error)"=w688, "State Machine.lvclass"=w690, "Device in"=w695) -> ("error out"=w694:errorcluster, "Device out"=w696:refnum<class "Trigger.lvclass">)  [unwired: 7 in]
              n255 = Increment(x=w693) -> (x+1=w686:u32)
              n256 = call-dynamic "Write Trigger.lvclass.vi"("error in (no error)"=w694, "Trigger.lvclass"=w696, "Sync Box in"=w702) -> ("error out"=w683:errorcluster, "Sync Box out"=w685:refnum<class "Sync Box.lvclass">)  [unwired: 7 in]
              n257 = call-dynamic "Write busy.vi"("error in (no error)"=w683, "busy"=TRUE, "Sync Box in"=w685) -> ("error out"=w682:errorcluster, "Sync Box out"=w684:refnum<class "Sync Box.lvclass">)  [unwired: 7 in]
            }
            frame True {
            }
          }
          n258 = call-dynamic "Write Sync Box.lvclass.vi"("error in (no error)"=w678, "Sync Box.lvclass"=w680, "SPARC4_AC in"=w679) -> ("error out"=w672:errorcluster, "SPARC4_AC out"=w674:refnum<class "S4ACS_GUI.lvclass">)  [unwired: 7 in]
          n259 = call-dynamic "Write Acq_state.vi"("error in (no error)"=w672, "Acq_state"=w673, "Acquisition in"=w669) -> ("error out"=w670:errorcluster, "Acquisition out"=w671:refnum<class "Acquisition.lvclass">)  [unwired: 7 in]
        }
        frame 305 {
          # "Espera terminar a execução do comando atual \nantes de ir ao proximo passo da Observação."
          n260 = call-dynamic "Read Sync Box.lvclass.vi"("error in (no error)"=w729, "SPARC4_AC in"=w730) -> ("error out"=w733:errorcluster, "Sync Box.lvclass"=w734:refnum<class "Sync Box.lvclass">, "SPARC4_AC out"=w731:refnum<class "S4ACS_GUI.lvclass">)  [unwired: 7 in]
          n261 = call-dynamic "Read Trigger.lvclass.vi"("error in (no error)"=w733, "Sync Box in"=w734) -> ("error out"=w728:errorcluster, "Trigger.lvclass"=w727:refnum<class "Trigger.lvclass">, "Sync Box out"=w732:refnum<class "Sync Box.lvclass">)  [unwired: 7 in]
          n262 = call-dynamic "Read State Machine.vi"("error in (no error)"=w728, "Device in"=w727) -> ("error out"=w721:errorcluster, "State Machine.lvclass"=w723:refnum<class "State Machine.lvclass">, "Device out"=w725:refnum<class "Trigger.lvclass">)  [unwired: 7 in]
          n263 = call-dynamic "Read State.vi"("error in (no error)"=w721, "State Machine in"=w723) -> ("error out"=w720:errorcluster, "State"=w719:i32, "State Machine out"=w722:refnum<class "State Machine.lvclass">)  [unwired: 7 in]
          n264 = Equal To 0?(x=w719) -> (x = 0?=w717:bool)
          n265 = call-dynamic "Write State Machine.vi"("error in (no error)"=w720, "State Machine.lvclass"=w722, "Device in"=w725) -> ("error out"=w724:errorcluster, "Device out"=w726:refnum<class "Trigger.lvclass">)  [unwired: 7 in]
          n266 = call-dynamic "Write Trigger.lvclass.vi"("error in (no error)"=w724, "Trigger.lvclass"=w726, "Sync Box in"=w732) -> ("error out"=w715:errorcluster, "Sync Box out"=w716:refnum<class "Sync Box.lvclass">)  [unwired: 7 in]
          n267 = case shown="True" w717 {
            tunnel: [w737 w743] -> w711
            tunnel: w718 -> [w737 w744]
            tunnel: w716 -> [w736 w742]
            tunnel: w715 -> [w735 w741]
            tunnel: [w735 w740] -> w714
            tunnel: [w736 w739] -> w713
            frame False {
            }
            frame True {
              # "Sinaliza que SyncBox\nficou livre."
              n268 = Increment(x=w744) -> (x+1=w743:u32)
              n269 = call-dynamic "Write busy.vi"("error in (no error)"=w741, "busy"=FALSE, "Sync Box in"=w742) -> ("error out"=w740:errorcluster, "Sync Box out"=w739:refnum<class "Sync Box.lvclass">)  [unwired: 7 in]
            }
          }
          n270 = call-dynamic "Write Sync Box.lvclass.vi"("error in (no error)"=w714, "Sync Box.lvclass"=w713, "SPARC4_AC in"=w731) -> ("error out"=w710:errorcluster, "SPARC4_AC out"=w712:refnum<class "S4ACS_GUI.lvclass">)  [unwired: 7 in]
          n271 = call-dynamic "Write Acq_state.vi"("error in (no error)"=w710, "Acq_state"=w711, "Acquisition in"=w709) -> ("error out"=w707:errorcluster, "Acquisition out"=w708:refnum<class "Acquisition.lvclass">)  [unwired: 7 in]
        }
        frame 306 {
          # "Dispara o comando para o dispositivo corrente."
          n272 = call-dynamic "Read Channel.vi"("error in (no error)"=w751, "Acquisition in"=w752) -> ("error out"=w763:errorcluster, "Channel.lvclass"=w762:refnum<class "Channel.lvclass">, "Acquisition out"=w767:refnum<class "Acquisition.lvclass">)  [unwired: 7 in]
          n273 = call-dynamic "Read State Machine.vi"("error in (no error)"=w763, "Device in"=w762) -> ("error out"=w764:errorcluster, "State Machine.lvclass"=w766:refnum<class "State Machine.lvclass">, "Device out"=w760:refnum<class "Channel.lvclass">)  [unwired: 7 in]
          n274 = call "Next State.vi"("error in (no error)"=w764, "New_State"=50, "State Machine in"=w766) -> ("error out"=w754:errorcluster, "State Machine out"=w756:refnum<class "State Machine.lvclass">)  [unwired: 7 in]
          n275 = call-dynamic "Write Timer.vi"("error in (no error)"=w754, "Timer"=u32 2, "State Machine in"=w756) -> ("error out"=w753:errorcluster, "State Machine out"=w755:refnum<class "State Machine.lvclass">)  [unwired: 7 in]
          n276 = call-dynamic "Write State Machine.vi"("error in (no error)"=w753, "State Machine.lvclass"=w755, "Device in"=w760) -> ("error out"=w759:errorcluster, "Device out"=w761:refnum<class "Channel.lvclass">)  [unwired: 7 in]
          n277 = Increment(x=w758) -> (x+1=w750:u32)
          n278 = call-dynamic "Write Channel.vi"("error in (no error)"=w759, "Channel.lvclass"=w761, "Acquisition in"=w767) -> ("error out"=w748:errorcluster, "Acquisition out"=w747:refnum<class "Acquisition.lvclass">)  [unwired: 7 in]
          n279 = call-dynamic "Write Acq_state.vi"("error in (no error)"=w748, "Acq_state"=w750, "Acquisition in"=w747) -> ("error out"=w745:errorcluster, "Acquisition out"=w746:refnum<class "Acquisition.lvclass">)  [unwired: 7 in]
        }
        frame 307 {
          # "Espera terminar a pausa carregada no Timer"
          n280 = call "Read Instrument.lvclass.vi"("error in (no error)"=w786, "S4ACS_GUI in"=w787) -> ("error out"=w792:errorcluster, "Instrument.lvclass"=w793:refnum<class "Instrument.lvclass">, "S4ACS_GUI out"=w789:refnum<class "S4ACS_GUI.lvclass">)  [unwired: 7 in]
          n281 = call "Read WPROT.vi"("error in (no error)"=w792, "Instrument in"=w793) -> ("error out"=w785:errorcluster, "Opt_Selector.lvclass"=w784:refnum<class "Opt_Selector.lvclass">, "Instrument out"=w791:refnum<class "Instrument.lvclass">)  [unwired: 7 in]
          n282 = call-dynamic "Read State Machine.vi"("error in (no error)"=w785, "Device in"=w784) -> ("error out"=w777:errorcluster, "State Machine.lvclass"=w778:refnum<class "State Machine.lvclass">, "Device out"=w782:refnum<class "Opt_Selector.lvclass">)  [unwired: 7 in]
          n283 = Increment(x=w774) -> (x+1=w779:u32)
          n284 = call "Verify Timer.vi"("error in (no error)"=w777, "State Machine in"=w778) -> ("error out"=w775:errorcluster, "timeout"=w780:bool, "State Machine out"=w776:refnum<class "State Machine.lvclass">)  [unwired: 7 in]
          n285 = call-dynamic "Write State Machine.vi"("error in (no error)"=w775, "State Machine.lvclass"=w776, "Device in"=w782) -> ("error out"=w781:errorcluster, "Device out"=w783:refnum<class "Opt_Selector.lvclass">)  [unwired: 7 in]
          n286 = call "Write WPROT.vi"("error in (no error)"=w781, "Opt_Selector.lvclass"=w783, "Instrument in"=w791) -> ("error out"=w788:errorcluster, "Instrument out"=w790:refnum<class "Instrument.lvclass">)  [unwired: 7 in]
          n287 = call "Write Instrument.lvclass.vi"("error in (no error)"=w788, "Instrument.lvclass"=w790, "S4ACS_GUI in"=w789) -> ("error out"=w770:errorcluster, "S4ACS_GUI out"=w773:refnum<class "S4ACS_GUI.lvclass">)  [unwired: 7 in]
          n288 = Select(t=w779, s=w780, f=w774) -> (s? t:f=w771:u32)
          n289 = call-dynamic "Write Acq_state.vi"("error in (no error)"=w770, "Acq_state"=w771, "Acquisition in"=w768) -> ("error out"=w769:errorcluster, "Acquisition out"=w772:refnum<class "Acquisition.lvclass">)  [unwired: 7 in]
        }
        frame 308 {
          n290 = call-dynamic "Read Sync Box.lvclass.vi"("error in (no error)"=w806, "SPARC4_AC in"=w807) -> ("error out"=w796:errorcluster, "Sync Box.lvclass"=w798:refnum<class "Sync Box.lvclass">, "SPARC4_AC out"=w809:refnum<class "S4ACS_GUI.lvclass">)  [unwired: 7 in]
          n291 = call-dynamic "Read busy.vi"("error in (no error)"=w796, "Sync Box in"=w798) -> ("error out"=w795:errorcluster, "busy"=w794:bool, "Sync Box out"=w797:refnum<class "Sync Box.lvclass">)  [unwired: 7 in]
          n292 = case shown="False" w794 {
            tunnel: w795 -> [w830 w832]
            tunnel: [w812 w833] -> w810
            tunnel: [w811 w832] -> w808
            tunnel: w805 -> [w820 w831]
            tunnel: w797 -> [w819 w833]
            tunnel: [w816 w831] -> w801
            frame False {
              # "Sinaliza que SyncBox\nestá ocupado."
              # "Dispara o comando para o dispositivo corrente."
              # "envia comando TRIGGER para o SyncBox"
              n293 = call-dynamic "Read Trigger.lvclass.vi"("error in (no error)"=w830, "Sync Box in"=w819) -> ("error out"=w825:errorcluster, "Trigger.lvclass"=w824:refnum<class "Trigger.lvclass">, "Sync Box out"=w829:refnum<class "Sync Box.lvclass">)  [unwired: 7 in]
              n294 = call-dynamic "Read State Machine.vi"("error in (no error)"=w825, "Device in"=w824) -> ("error out"=w826:errorcluster, "State Machine.lvclass"=w828:refnum<class "State Machine.lvclass">, "Device out"=w822:refnum<class "Trigger.lvclass">)  [unwired: 7 in]
              n295 = call "Next State.vi"("error in (no error)"=w826, "New_State"=30, "State Machine in"=w828) -> ("error out"=w817:errorcluster, "State Machine out"=w818:refnum<class "State Machine.lvclass">)  [unwired: 7 in]
              n296 = call-dynamic "Write State Machine.vi"("error in (no error)"=w817, "State Machine.lvclass"=w818, "Device in"=w822) -> ("error out"=w821:errorcluster, "Device out"=w823:refnum<class "Trigger.lvclass">)  [unwired: 7 in]
              n297 = call-dynamic "Write Trigger.lvclass.vi"("error in (no error)"=w821, "Trigger.lvclass"=w823, "Sync Box in"=w829) -> ("error out"=w814:errorcluster, "Sync Box out"=w815:refnum<class "Sync Box.lvclass">)  [unwired: 7 in]
              n298 = Increment(x=w820) -> (x+1=w816:u32)
              n299 = call-dynamic "Write busy.vi"("error in (no error)"=w814, "busy"=TRUE, "Sync Box in"=w815) -> ("error out"=w811:errorcluster, "Sync Box out"=w812:refnum<class "Sync Box.lvclass">)  [unwired: 7 in]
            }
            frame True {
            }
          }
          n300 = call-dynamic "Write Sync Box.lvclass.vi"("error in (no error)"=w808, "Sync Box.lvclass"=w810, "SPARC4_AC in"=w809) -> ("error out"=w802:errorcluster, "SPARC4_AC out"=w804:refnum<class "S4ACS_GUI.lvclass">)  [unwired: 7 in]
          n301 = call-dynamic "Write Acq_state.vi"("error in (no error)"=w802, "Acq_state"=w801, "Acquisition in"=w800) -> ("error out"=w799:errorcluster, "Acquisition out"=w803:refnum<class "Acquisition.lvclass">)  [unwired: 7 in]
        }
        frame 309 {
          # "Espera terminar a execução do comando atual \nantes de ir ao proximo passo da Observação."
          n302 = call-dynamic "Read Sync Box.lvclass.vi"("error in (no error)"=w856, "SPARC4_AC in"=w857) -> ("error out"=w860:errorcluster, "Sync Box.lvclass"=w861:refnum<class "Sync Box.lvclass">, "SPARC4_AC out"=w858:refnum<class "S4ACS_GUI.lvclass">)  [unwired: 7 in]
          n303 = call-dynamic "Read Trigger.lvclass.vi"("error in (no error)"=w860, "Sync Box in"=w861) -> ("error out"=w855:errorcluster, "Trigger.lvclass"=w854:refnum<class "Trigger.lvclass">, "Sync Box out"=w859:refnum<class "Sync Box.lvclass">)  [unwired: 7 in]
          n304 = call-dynamic "Read State Machine.vi"("error in (no error)"=w855, "Device in"=w854) -> ("error out"=w848:errorcluster, "State Machine.lvclass"=w850:refnum<class "State Machine.lvclass">, "Device out"=w852:refnum<class "Trigger.lvclass">)  [unwired: 7 in]
          n305 = call-dynamic "Read State.vi"("error in (no error)"=w848, "State Machine in"=w850) -> ("error out"=w847:errorcluster, "State"=w846:i32, "State Machine out"=w849:refnum<class "State Machine.lvclass">)  [unwired: 7 in]
          n306 = Equal To 0?(x=w846) -> (x = 0?=w840:bool)
          n307 = call-dynamic "Write State Machine.vi"("error in (no error)"=w847, "State Machine.lvclass"=w849, "Device in"=w852) -> ("error out"=w851:errorcluster, "Device out"=w853:refnum<class "Trigger.lvclass">)  [unwired: 7 in]
          n308 = call-dynamic "Write Trigger.lvclass.vi"("error in (no error)"=w851, "Trigger.lvclass"=w853, "Sync Box in"=w859) -> ("error out"=w838:errorcluster, "Sync Box out"=w839:refnum<class "Sync Box.lvclass">)  [unwired: 7 in]
          n309 = case shown="True" w840 {
            tunnel: w845 -> [w862 w871]
            tunnel: w839 -> [w864 w870]
            tunnel: w838 -> [w863 w869]
            tunnel: [w863 w868] -> w837
            tunnel: [w864 w867] -> w836
            tunnel: [w862 w865] -> w835
            frame False {
            }
            frame True {
              # "Sinaliza que SyncBox\nestá livre."
              n310 = call-dynamic "Write busy.vi"("error in (no error)"=w869, "busy"=FALSE, "Sync Box in"=w870) -> ("error out"=w868:errorcluster, "Sync Box out"=w867:refnum<class "Sync Box.lvclass">)  [unwired: 7 in]
              n311 = Increment(x=w871) -> (x+1=w865:u32)
            }
          }
          n312 = call-dynamic "Write Sync Box.lvclass.vi"("error in (no error)"=w837, "Sync Box.lvclass"=w836, "SPARC4_AC in"=w858) -> ("error out"=w843:errorcluster, "SPARC4_AC out"=w844:refnum<class "S4ACS_GUI.lvclass">)  [unwired: 7 in]
          n313 = call-dynamic "Write Acq_state.vi"("error in (no error)"=w843, "Acq_state"=w835, "Acquisition in"=w834) -> ("error out"=w841:errorcluster, "Acquisition out"=w842:refnum<class "Acquisition.lvclass">)  [unwired: 7 in]
        }
        frame 310 {
          # "Espera terminar a execução do comando atual \nantes de ir ao proximo passo da Observação."
          n314 = call-dynamic "Read Channel.vi"("error in (no error)"=w878, "Acquisition in"=w879) -> ("error out"=w892:errorcluster, "Channel.lvclass"=w891:refnum<class "Channel.lvclass">, "Acquisition out"=w893:refnum<class "Acquisition.lvclass">)  [unwired: 7 in]
          n315 = call-dynamic "Read State Machine.vi"("error in (no error)"=w892, "Device in"=w891) -> ("error out"=w885:errorcluster, "State Machine.lvclass"=w887:refnum<class "State Machine.lvclass">, "Device out"=w889:refnum<class "Channel.lvclass">)  [unwired: 7 in]
          n316 = call-dynamic "Read State.vi"("error in (no error)"=w885, "State Machine in"=w887) -> ("error out"=w884:errorcluster, "State"=w882:i32, "State Machine out"=w886:refnum<class "State Machine.lvclass">)  [unwired: 7 in]
          n317 = call-dynamic "Write State Machine.vi"("error in (no error)"=w884, "State Machine.lvclass"=w886, "Device in"=w889) -> ("error out"=w888:errorcluster, "Device out"=w890:refnum<class "Channel.lvclass">)  [unwired: 7 in]
          n318 = Equal To 0?(x=w882) -> (x = 0?=w883:bool)
          n319 = call-dynamic "Write Channel.vi"("error in (no error)"=w888, "Channel.lvclass"=w890, "Acquisition in"=w893) -> ("error out"=w875:errorcluster, "Acquisition out"=w877:refnum<class "Acquisition.lvclass">)  [unwired: 7 in]
          n320 = Select(t=u32 301, s=w883, f=w881) -> (s? t:f=w876:u32)
          n321 = call-dynamic "Write Acq_state.vi"("error in (no error)"=w875, "Acq_state"=w876, "Acquisition in"=w877) -> ("error out"=w872:errorcluster, "Acquisition out"=w873:refnum<class "Acquisition.lvclass">)  [unwired: 7 in]
        }
        frame 311 {
          n322 = call-dynamic "Read Channel.vi"("error in (no error)"=w910, "Acquisition in"=w909) -> ("error out"=w908:errorcluster, "Channel.lvclass"=w907:refnum<class "Channel.lvclass">, "Acquisition out"=w894:refnum<class "Acquisition.lvclass">)  [unwired: 7 in]
          n323 = call-dynamic "Read ciclos.vi"("error in (no error)"=w908, "Channel in"=w907) -> ("error out"=w904:errorcluster, "ciclos"=w906:u32, "Channel out"=w895:refnum<class "Channel.lvclass">)  [unwired: 7 in]
          n324 = Decrement(x=w906) -> (x-1=w911:u32)
          n325 = Greater Than 0?(x=w911) -> (x > 0?=w915:bool)
          n326 = case shown="True" w915 {
            selector: w915 -> [w917 w919]
            tunnel: w911 -> [_ w918]
            tunnel: [w917 w919] -> w914
            tunnel: [u32 0 w918] -> w900
            frame False {
            }
            frame True {
            }
          }
          n327 = call-dynamic "Write ciclos.vi"("error in (no error)"=w904, "ciclos"=w900, "Channel in"=w895) -> ("error out"=w902:errorcluster, "Channel out"=w901:refnum<class "Channel.lvclass">)  [unwired: 7 in]
          n328 = Select(t=u32 301, s=w914, f=u32 0) -> (s? t:f=w905:u32)
          n329 = call-dynamic "Write Channel.vi"("error in (no error)"=w902, "Channel.lvclass"=w901, "Acquisition in"=w894) -> ("error out"=w898:errorcluster, "Acquisition out"=w899:refnum<class "Acquisition.lvclass">)  [unwired: 7 in]
          n330 = call-dynamic "Write Acq_state.vi"("error in (no error)"=w898, "Acq_state"=w905, "Acquisition in"=w899) -> ("error out"=w896:errorcluster, "Acquisition out"=w897:refnum<class "Acquisition.lvclass">)  [unwired: 7 in]
        }
        frame 321 {
          n331 = call-dynamic "Read Sync Box.lvclass.vi"("error in (no error)"=w932, "SPARC4_AC in"=w933) -> ("error out"=w923:errorcluster, "Sync Box.lvclass"=w924:refnum<class "Sync Box.lvclass">, "SPARC4_AC out"=w935:refnum<class "S4ACS_GUI.lvclass">)  [unwired: 7 in]
          n332 = call-dynamic "Read busy.vi"("error in (no error)"=w923, "Sync Box in"=w924) -> ("error out"=w920:errorcluster, "busy"=w922:bool, "Sync Box out"=w921:refnum<class "Sync Box.lvclass">)  [unwired: 7 in]
          n333 = case shown="False" w922 {
            tunnel: [w940 w962] -> w936
            tunnel: [w938 w961] -> w934
            tunnel: w931 -> [w950 w960]
            tunnel: [w944 w960] -> w927
            tunnel: w921 -> [w943 w962]
            tunnel: w920 -> [w942 w961]
            frame False {
              # "configura delays do syncBox"
              # "Dispara o comando para o dispositivo corrente."
              n334 = call-dynamic "Read Trigger.lvclass.vi"("error in (no error)"=w942, "Sync Box in"=w943) -> ("error out"=w955:errorcluster, "Trigger.lvclass"=w954:refnum<class "Trigger.lvclass">, "Sync Box out"=w959:refnum<class "Sync Box.lvclass">)  [unwired: 7 in]
              n335 = call-dynamic "Read State Machine.vi"("error in (no error)"=w955, "Device in"=w954) -> ("error out"=w956:errorcluster, "State Machine.lvclass"=w958:refnum<class "State Machine.lvclass">, "Device out"=w952:refnum<class "Trigger.lvclass">)  [unwired: 7 in]
              n336 = call "Next State.vi"("error in (no error)"=w956, "New_State"=10, "State Machine in"=w958) -> ("error out"=w946:errorcluster, "State Machine out"=w948:refnum<class "State Machine.lvclass">)  [unwired: 7 in]
              n337 = call-dynamic "Write Timer.vi"("error in (no error)"=w946, "Timer"=u32 5, "State Machine in"=w948) -> ("error out"=w945:errorcluster, "State Machine out"=w947:refnum<class "State Machine.lvclass">)  [unwired: 7 in]
              n338 = call-dynamic "Write State Machine.vi"("error in (no error)"=w945, "State Machine.lvclass"=w947, "Device in"=w952) -> ("error out"=w951:errorcluster, "Device out"=w953:refnum<class "Trigger.lvclass">)  [unwired: 7 in]
              n339 = call-dynamic "Write Trigger.lvclass.vi"("error in (no error)"=w951, "Trigger.lvclass"=w953, "Sync Box in"=w959) -> ("error out"=w939:errorcluster, "Sync Box out"=w941:refnum<class "Sync Box.lvclass">)  [unwired: 7 in]
              n340 = Increment(x=w950) -> (x+1=w944:u32)
              n341 = call-dynamic "Write busy.vi"("error in (no error)"=w939, "busy"=TRUE, "Sync Box in"=w941) -> ("error out"=w938:errorcluster, "Sync Box out"=w940:refnum<class "Sync Box.lvclass">)  [unwired: 7 in]
            }
            frame True {
            }
          }
          n342 = call-dynamic "Write Sync Box.lvclass.vi"("error in (no error)"=w934, "Sync Box.lvclass"=w936, "SPARC4_AC in"=w935) -> ("error out"=w928:errorcluster, "SPARC4_AC out"=w930:refnum<class "S4ACS_GUI.lvclass">)  [unwired: 7 in]
          n343 = call-dynamic "Write Acq_state.vi"("error in (no error)"=w928, "Acq_state"=w927, "Acquisition in"=w926) -> ("error out"=w925:errorcluster, "Acquisition out"=w929:refnum<class "Acquisition.lvclass">)  [unwired: 7 in]
        }
        frame 322 {
          # "Espera terminar a execução do comando atual \nantes de ir ao proximo passo da Observação."
          n344 = call-dynamic "Read Sync Box.lvclass.vi"("error in (no error)"=w985, "SPARC4_AC in"=w986) -> ("error out"=w989:errorcluster, "Sync Box.lvclass"=w990:refnum<class "Sync Box.lvclass">, "SPARC4_AC out"=w987:refnum<class "S4ACS_GUI.lvclass">)  [unwired: 7 in]
          n345 = call-dynamic "Read Trigger.lvclass.vi"("error in (no error)"=w989, "Sync Box in"=w990) -> ("error out"=w984:errorcluster, "Trigger.lvclass"=w983:refnum<class "Trigger.lvclass">, "Sync Box out"=w988:refnum<class "Sync Box.lvclass">)  [unwired: 7 in]
          n346 = call-dynamic "Read State Machine.vi"("error in (no error)"=w984, "Device in"=w983) -> ("error out"=w977:errorcluster, "State Machine.lvclass"=w979:refnum<class "State Machine.lvclass">, "Device out"=w981:refnum<class "Trigger.lvclass">)  [unwired: 7 in]
          n347 = call-dynamic "Read State.vi"("error in (no error)"=w977, "State Machine in"=w979) -> ("error out"=w976:errorcluster, "State"=w975:i32, "State Machine out"=w978:refnum<class "State Machine.lvclass">)  [unwired: 7 in]
          n348 = Equal To 0?(x=w975) -> (x = 0?=w963:bool)
          n349 = call-dynamic "Write State Machine.vi"("error in (no error)"=w976, "State Machine.lvclass"=w978, "Device in"=w981) -> ("error out"=w980:errorcluster, "Device out"=w982:refnum<class "Trigger.lvclass">)  [unwired: 7 in]
          n350 = call-dynamic "Write Trigger.lvclass.vi"("error in (no error)"=w980, "Trigger.lvclass"=w982, "Sync Box in"=w988) -> ("error out"=w965:errorcluster, "Sync Box out"=w967:refnum<class "Sync Box.lvclass">)  [unwired: 7 in]
          n351 = case shown="True" w963 {
            tunnel: w974 -> [w993 w1000]
            tunnel: [w993 w999] -> w968
            tunnel: [w992 w997] -> w966
            tunnel: w967 -> [w992 w998]
            tunnel: [w991 w995] -> w964
            tunnel: w965 -> [w991 w996]
            frame False {
            }
            frame True {
              n352 = call-dynamic "Write busy.vi"("error in (no error)"=w996, "busy"=FALSE, "Sync Box in"=w998) -> ("error out"=w995:errorcluster, "Sync Box out"=w997:refnum<class "Sync Box.lvclass">)  [unwired: 7 in]
              n353 = Increment(x=w1000) -> (x+1=w999:u32)
            }
          }
          n354 = call-dynamic "Write Sync Box.lvclass.vi"("error in (no error)"=w964, "Sync Box.lvclass"=w966, "SPARC4_AC in"=w987) -> ("error out"=w971:errorcluster, "SPARC4_AC out"=w973:refnum<class "S4ACS_GUI.lvclass">)  [unwired: 7 in]
          n355 = call-dynamic "Write Acq_state.vi"("error in (no error)"=w971, "Acq_state"=w968, "Acquisition in"=w969) -> ("error out"=w970:errorcluster, "Acquisition out"=w972:refnum<class "Acquisition.lvclass">)  [unwired: 7 in]
        }
        frame 323 {
          # "Dispara o comando para o dispositivo corrente."
          n356 = call-dynamic "Read Channel.vi"("error in (no error)"=w1007, "Acquisition in"=w1008) -> ("error out"=w1019:errorcluster, "Channel.lvclass"=w1018:refnum<class "Channel.lvclass">, "Acquisition out"=w1023:refnum<class "Acquisition.lvclass">)  [unwired: 7 in]
          n357 = call-dynamic "Read State Machine.vi"("error in (no error)"=w1019, "Device in"=w1018) -> ("error out"=w1020:errorcluster, "State Machine.lvclass"=w1022:refnum<class "State Machine.lvclass">, "Device out"=w1016:refnum<class "Channel.lvclass">)  [unwired: 7 in]
          n358 = call "Next State.vi"("error in (no error)"=w1020, "New_State"=50, "State Machine in"=w1022) -> ("error out"=w1010:errorcluster, "State Machine out"=w1012:refnum<class "State Machine.lvclass">)  [unwired: 7 in]
          n359 = call-dynamic "Write Timer.vi"("error in (no error)"=w1010, "Timer"=u32 2, "State Machine in"=w1012) -> ("error out"=w1009:errorcluster, "State Machine out"=w1011:refnum<class "State Machine.lvclass">)  [unwired: 7 in]
          n360 = call-dynamic "Write State Machine.vi"("error in (no error)"=w1009, "State Machine.lvclass"=w1011, "Device in"=w1016) -> ("error out"=w1015:errorcluster, "Device out"=w1017:refnum<class "Channel.lvclass">)  [unwired: 7 in]
          n361 = Increment(x=w1014) -> (x+1=w1004:u32)
          n362 = call-dynamic "Write Channel.vi"("error in (no error)"=w1015, "Channel.lvclass"=w1017, "Acquisition in"=w1023) -> ("error out"=w1003:errorcluster, "Acquisition out"=w1005:refnum<class "Acquisition.lvclass">)  [unwired: 7 in]
          n363 = call-dynamic "Write Acq_state.vi"("error in (no error)"=w1003, "Acq_state"=w1004, "Acquisition in"=w1005) -> ("error out"=w1001:errorcluster, "Acquisition out"=w1006:refnum<class "Acquisition.lvclass">)  [unwired: 7 in]
        }
        frame 324 {
          n364 = call-dynamic "Read Sync Box.lvclass.vi"("error in (no error)"=w1036, "SPARC4_AC in"=w1037) -> ("error out"=w1031:errorcluster, "Sync Box.lvclass"=w1034:refnum<class "Sync Box.lvclass">, "SPARC4_AC out"=w1039:refnum<class "S4ACS_GUI.lvclass">)  [unwired: 7 in]
          n365 = call-dynamic "Read busy.vi"("error in (no error)"=w1031, "Sync Box in"=w1034) -> ("error out"=w1030:errorcluster, "busy"=w1033:bool, "Sync Box out"=w1032:refnum<class "Sync Box.lvclass">)  [unwired: 7 in]
          n366 = case shown="True" w1033 {
            tunnel: w1030 -> [w1060 w1062]
            tunnel: [w1044 w1063] -> w1040
            tunnel: [w1042 w1062] -> w1038
            tunnel: w1035 -> [w1050 w1061]
            tunnel: [w1049 w1061] -> w1028
            tunnel: w1032 -> [w1048 w1063]
            frame False {
              # "envia comando TRIGGER para o SyncBox"
              # "Dispara o comando para o dispositivo corrente."
              n367 = call-dynamic "Read Trigger.lvclass.vi"("error in (no error)"=w1060, "Sync Box in"=w1048) -> ("error out"=w1055:errorcluster, "Trigger.lvclass"=w1054:refnum<class "Trigger.lvclass">, "Sync Box out"=w1059:refnum<class "Sync Box.lvclass">)  [unwired: 7 in]
              n368 = call-dynamic "Read State Machine.vi"("error in (no error)"=w1055, "Device in"=w1054) -> ("error out"=w1056:errorcluster, "State Machine.lvclass"=w1058:refnum<class "State Machine.lvclass">, "Device out"=w1052:refnum<class "Trigger.lvclass">)  [unwired: 7 in]
              n369 = call "Next State.vi"("error in (no error)"=w1056, "New_State"=30, "State Machine in"=w1058) -> ("error out"=w1046:errorcluster, "State Machine out"=w1047:refnum<class "State Machine.lvclass">)  [unwired: 7 in]
              n370 = call-dynamic "Write State Machine.vi"("error in (no error)"=w1046, "State Machine.lvclass"=w1047, "Device in"=w1052) -> ("error out"=w1051:errorcluster, "Device out"=w1053:refnum<class "Trigger.lvclass">)  [unwired: 7 in]
              n371 = Increment(x=w1050) -> (x+1=w1049:u32)
              n372 = call-dynamic "Write Trigger.lvclass.vi"("error in (no error)"=w1051, "Trigger.lvclass"=w1053, "Sync Box in"=w1059) -> ("error out"=w1043:errorcluster, "Sync Box out"=w1045:refnum<class "Sync Box.lvclass">)  [unwired: 7 in]
              n373 = call-dynamic "Write busy.vi"("error in (no error)"=w1043, "busy"=TRUE, "Sync Box in"=w1045) -> ("error out"=w1042:errorcluster, "Sync Box out"=w1044:refnum<class "Sync Box.lvclass">)  [unwired: 7 in]
            }
            frame True {
            }
          }
          n374 = call-dynamic "Write Sync Box.lvclass.vi"("error in (no error)"=w1038, "Sync Box.lvclass"=w1040, "SPARC4_AC in"=w1039) -> ("error out"=w1027:errorcluster, "SPARC4_AC out"=w1029:refnum<class "S4ACS_GUI.lvclass">)  [unwired: 7 in]
          n375 = call-dynamic "Write Acq_state.vi"("error in (no error)"=w1027, "Acq_state"=w1028, "Acquisition in"=w1024) -> ("error out"=w1026:errorcluster, "Acquisition out"=w1025:refnum<class "Acquisition.lvclass">)  [unwired: 7 in]
        }
        frame 325 {
          # "Espera terminar a execução do comando atual \nantes de ir ao proximo passo da Observação."
          n376 = call-dynamic "Read Sync Box.lvclass.vi"("error in (no error)"=w1086, "SPARC4_AC in"=w1087) -> ("error out"=w1090:errorcluster, "Sync Box.lvclass"=w1091:refnum<class "Sync Box.lvclass">, "SPARC4_AC out"=w1088:refnum<class "S4ACS_GUI.lvclass">)  [unwired: 7 in]
          n377 = call-dynamic "Read Trigger.lvclass.vi"("error in (no error)"=w1090, "Sync Box in"=w1091) -> ("error out"=w1085:errorcluster, "Trigger.lvclass"=w1084:refnum<class "Trigger.lvclass">, "Sync Box out"=w1089:refnum<class "Sync Box.lvclass">)  [unwired: 7 in]
          n378 = call-dynamic "Read State Machine.vi"("error in (no error)"=w1085, "Device in"=w1084) -> ("error out"=w1078:errorcluster, "State Machine.lvclass"=w1080:refnum<class "State Machine.lvclass">, "Device out"=w1082:refnum<class "Trigger.lvclass">)  [unwired: 7 in]
          n379 = call-dynamic "Read State.vi"("error in (no error)"=w1078, "State Machine in"=w1080) -> ("error out"=w1077:errorcluster, "State"=w1076:i32, "State Machine out"=w1079:refnum<class "State Machine.lvclass">)  [unwired: 7 in]
          n380 = Equal To 0?(x=w1076) -> (x = 0?=w1070:bool)
          n381 = call-dynamic "Write State Machine.vi"("error in (no error)"=w1077, "State Machine.lvclass"=w1079, "Device in"=w1082) -> ("error out"=w1081:errorcluster, "Device out"=w1083:refnum<class "Trigger.lvclass">)  [unwired: 7 in]
          n382 = call-dynamic "Write Trigger.lvclass.vi"("error in (no error)"=w1081, "Trigger.lvclass"=w1083, "Sync Box in"=w1089) -> ("error out"=w1068:errorcluster, "Sync Box out"=w1069:refnum<class "Sync Box.lvclass">)  [unwired: 7 in]
          n383 = case shown="True" w1070 {
            tunnel: w1075 -> [w1092 w1101]
            tunnel: [w1094 w1099] -> w1066
            tunnel: w1069 -> [w1094 w1100]
            tunnel: [w1093 w1097] -> w1067
            tunnel: w1068 -> [w1093 w1098]
            tunnel: [w1092 w1096] -> w1065
            frame False {
            }
            frame True {
              n384 = Increment(x=w1101) -> (x+1=w1096:u32)
              n385 = call-dynamic "Write busy.vi"("error in (no error)"=w1098, "busy"=FALSE, "Sync Box in"=w1100) -> ("error out"=w1097:errorcluster, "Sync Box out"=w1099:refnum<class "Sync Box.lvclass">)  [unwired: 7 in]
            }
          }
          n386 = call-dynamic "Write Sync Box.lvclass.vi"("error in (no error)"=w1067, "Sync Box.lvclass"=w1066, "SPARC4_AC in"=w1088) -> ("error out"=w1073:errorcluster, "SPARC4_AC out"=w1074:refnum<class "S4ACS_GUI.lvclass">)  [unwired: 7 in]
          n387 = call-dynamic "Write Acq_state.vi"("error in (no error)"=w1073, "Acq_state"=w1065, "Acquisition in"=w1064) -> ("error out"=w1071:errorcluster, "Acquisition out"=w1072:refnum<class "Acquisition.lvclass">)  [unwired: 7 in]
        }
        frame 326 {
          # "Espera terminar a execução do comando atual \nantes de ir ao proximo passo da Observação."
          n388 = call-dynamic "Read Channel.vi"("error in (no error)"=w1103, "Acquisition in"=w1102) -> ("error out"=w1122:errorcluster, "Channel.lvclass"=w1121:refnum<class "Channel.lvclass">, "Acquisition out"=w1123:refnum<class "Acquisition.lvclass">)  [unwired: 7 in]
          n389 = call-dynamic "Read State Machine.vi"("error in (no error)"=w1122, "Device in"=w1121) -> ("error out"=w1115:errorcluster, "State Machine.lvclass"=w1117:refnum<class "State Machine.lvclass">, "Device out"=w1119:refnum<class "Channel.lvclass">)  [unwired: 7 in]
          n390 = call-dynamic "Read State.vi"("error in (no error)"=w1115, "State Machine in"=w1117) -> ("error out"=w1114:errorcluster, "State"=w1112:i32, "State Machine out"=w1116:refnum<class "State Machine.lvclass">)  [unwired: 7 in]
          n391 = Equal To 0?(x=w1112) -> (x = 0?=w1113:bool)
          n392 = call-dynamic "Write State Machine.vi"("error in (no error)"=w1114, "State Machine.lvclass"=w1116, "Device in"=w1119) -> ("error out"=w1118:errorcluster, "Device out"=w1120:refnum<class "Channel.lvclass">)  [unwired: 7 in]
          n393 = call-dynamic "Write Channel.vi"("error in (no error)"=w1118, "Channel.lvclass"=w1120, "Acquisition in"=w1123) -> ("error out"=w1105:errorcluster, "Acquisition out"=w1106:refnum<class "Acquisition.lvclass">)  [unwired: 7 in]
          n394 = Increment(x=w1111) -> (x+1=w1110:u32)
          n395 = Select(t=w1110, s=w1113, f=w1111) -> (s? t:f=w1108:u32)
          n396 = call-dynamic "Write Acq_state.vi"("error in (no error)"=w1105, "Acq_state"=w1108, "Acquisition in"=w1106) -> ("error out"=w1107:errorcluster, "Acquisition out"=w1109:refnum<class "Acquisition.lvclass">)  [unwired: 7 in]
        }
        frame 327 {
          n397 = call-dynamic "Read Channel.vi"("error in (no error)"=w1139, "Acquisition in"=w1140) -> ("error out"=w1137:errorcluster, "Channel.lvclass"=w1138:refnum<class "Channel.lvclass">, "Acquisition out"=w1133:refnum<class "Acquisition.lvclass">)  [unwired: 7 in]
          n398 = call-dynamic "Read ciclos.vi"("error in (no error)"=w1137, "Channel in"=w1138) -> ("error out"=w1128:errorcluster, "ciclos"=w1136:u32, "Channel out"=w1129:refnum<class "Channel.lvclass">)  [unwired: 7 in]
          n399 = Decrement(x=w1136) -> (x-1=w1141:u32)
          n400 = Greater Than 0?(x=w1141) -> (x > 0?=w1145:bool)
          n401 = case shown="True" w1145 {
            selector: w1145 -> [w1147 w1149]
            tunnel: w1141 -> [_ w1148]
            tunnel: [w1147 w1149] -> w1144
            tunnel: [u32 0 w1148] -> w1134
            frame False {
            }
            frame True {
            }
          }
          n402 = call-dynamic "Write ciclos.vi"("error in (no error)"=w1128, "ciclos"=w1134, "Channel in"=w1129) -> ("error out"=w1127:errorcluster, "Channel out"=w1130:refnum<class "Channel.lvclass">)  [unwired: 7 in]
          n403 = call-dynamic "Write Channel.vi"("error in (no error)"=w1127, "Channel.lvclass"=w1130, "Acquisition in"=w1133) -> ("error out"=w1126:errorcluster, "Acquisition out"=w1132:refnum<class "Acquisition.lvclass">)  [unwired: 7 in]
          n404 = Select(t=u32 321, s=w1144, f=u32 0) -> (s? t:f=w1124:u32)
          n405 = call-dynamic "Write Acq_state.vi"("error in (no error)"=w1126, "Acq_state"=w1124, "Acquisition in"=w1132) -> ("error out"=w1125:errorcluster, "Acquisition out"=w1131:refnum<class "Acquisition.lvclass">)  [unwired: 7 in]
        }
        frame 400 {
          # "Estado de \"Pause\": fica parado aqui até o botão START seja pressionado."
        }
      }
    }
    frame Error {
    }
  }
  "error out" <- w5
  "S4ACS_GUI out" <- w3
  "Acquisition.lvclass Out" <- w1
